vi "Client.vi"() -> ()   [LabVIEW 2021]
uses:
  <vilib>/Utility/file.llb/Write Delimited Spreadsheet (string).vi
panel:
  in  "Electric":dbl
  in  "Smart Home Control":T1(tab)
  out "Boolean":bool
  in  "Username":string
  in  "Password":string
  in  "Login":bool
  in  "AddUser":bool
  in  "DeleteUser":bool
  in  "Logout":bool
  out "Boolean2":bool
  out "LightSensor":bool
  in  "MasterBedroomL1":bool
  in  "MasterBedroomL2":bool
  in  "KitchenToiletL":bool
  in  "KitchenL":bool
  in  "LRToiletL":bool
  in  "LivingRoomL2":bool
  in  "LivingRoomL1":bool
  in  "BalconyL3":bool
  in  "BalconyL2":bool
  in  "BalconyL1":bool
  in  "Bedroom2L":bool
  in  "Bedroom1L":bool
  in  "OffL":bool
  in  "MBToiletDC":bool
  in  "MBToiletDO":bool
  in  "Bedroom2DO":bool
  in  "Bedroom2DC":bool
  out "DoorSensor":bool
  in  "Bedroom1DO":bool
  in  "Bedroom1DC":bool
  in  "MasterBedroomDC":bool
  in  "MasterBedroomDO":bool
  in  "KitchenDO":bool
  in  "KitchenDC":bool
  in  "KitchenToiletDO":bool
  in  "KitchenToiletDC":bool
  in  "LRToiletDC":bool
  in  "LRToiletDO":bool
  in  "LivingRoomDC":bool
  in  "LivingRoomDO":bool
  in  "Balcony2DC":bool
  in  "Balcony2DO":bool
  in  "Balcony1DO1":bool
  in  "Balcony1DC1":bool
  in  "Balcony1DO2":bool
  in  "Balcony1DC2":bool
  in  "OpenD":bool
  in  "CloseD":bool
  in  "MasterBedroomC":dbl(knob) scale=0.0..10.0
  in  "LivingRoomC":dbl(knob) scale=0.0..10.0
  in  "Pause":bool
  in  "Play":bool
  out "TVSensor":bool
  in  "Channel1":bool
  in  "Channel2":bool
  in  "Channel3":bool
  in  "Volume":dbl(knob) scale=0.0..100.0
  in  "Power":bool
  in  "Table Control":string[][](table)
  # "Smart Home Control System"
  # "Off All Lights"
  # "Bedroom 1"
  # "Bedroom 2"
  # "Living Room"
  # "Master Bedroom"
  # "Balcony 1"
  # "Kitchen"
  # "Master Bedroom"
  # "Kitchen"
  # "Living Room"
  # "Toilet"
  # "Toilet"
  # "Toilet"
  # "Bedroom 1"
  # "Balcony 1 to Master"
  # "Balcony 2"
  # "Bedroom 2"
  # "Balcony 1 to Kitchen"
  # "Open All"
  # "Close All"
  # "Master Bedroom"
  # "Living Room"
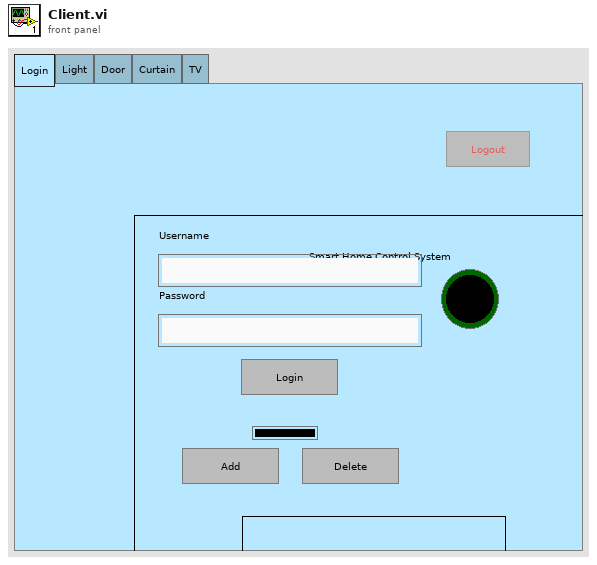
[diagram p1: front panel]
types:
  T1 = enum32{"Login", "Light", "Door", "Curtain", "TV"}
  T2 = enum32{"Page Enabled", "Page Disabled", "Page Disabled & Grayed"}
  T3 = enum8{"Enabled", "Disabled", "Disabled and Grayed Out"}
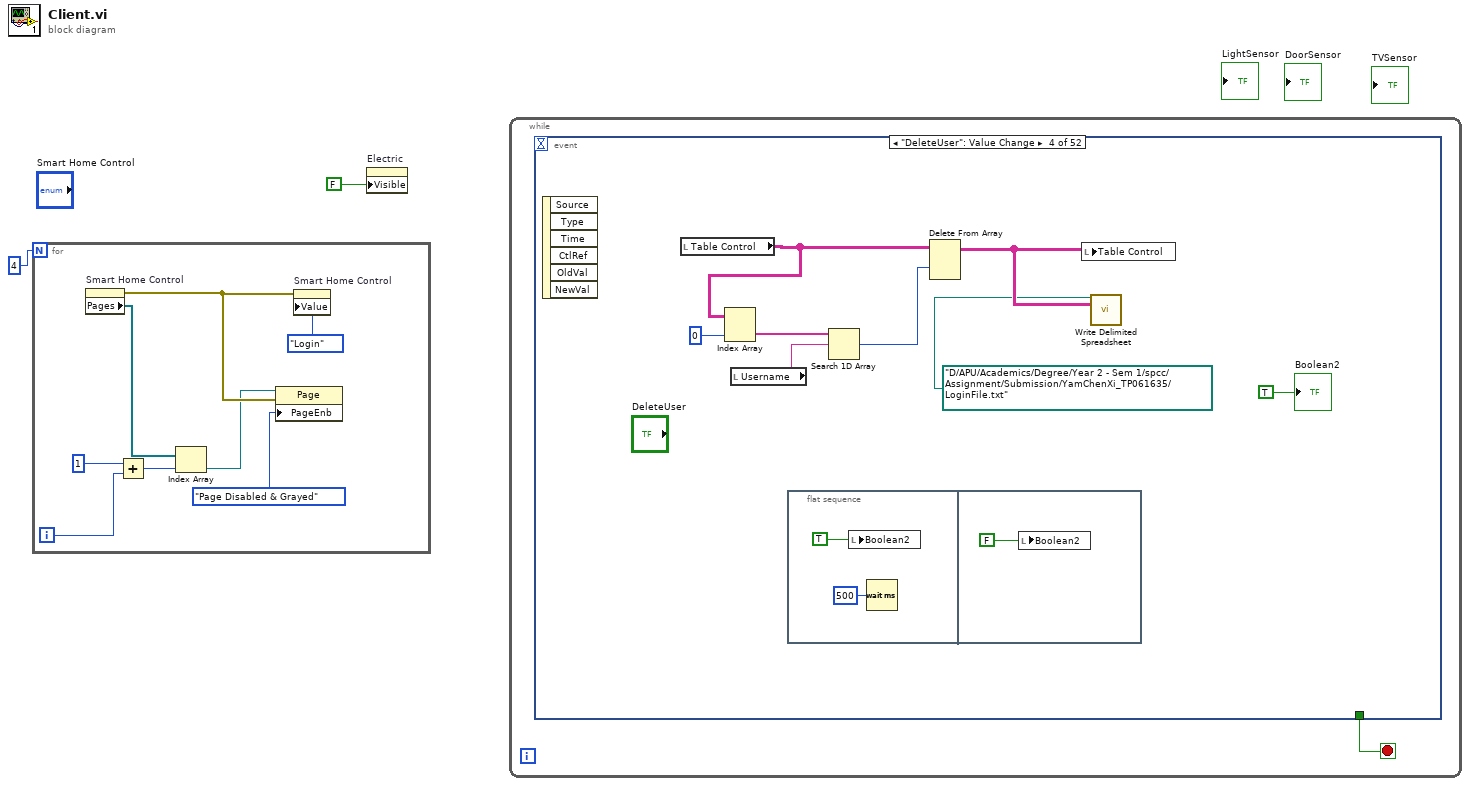
[diagram p0: block diagram]
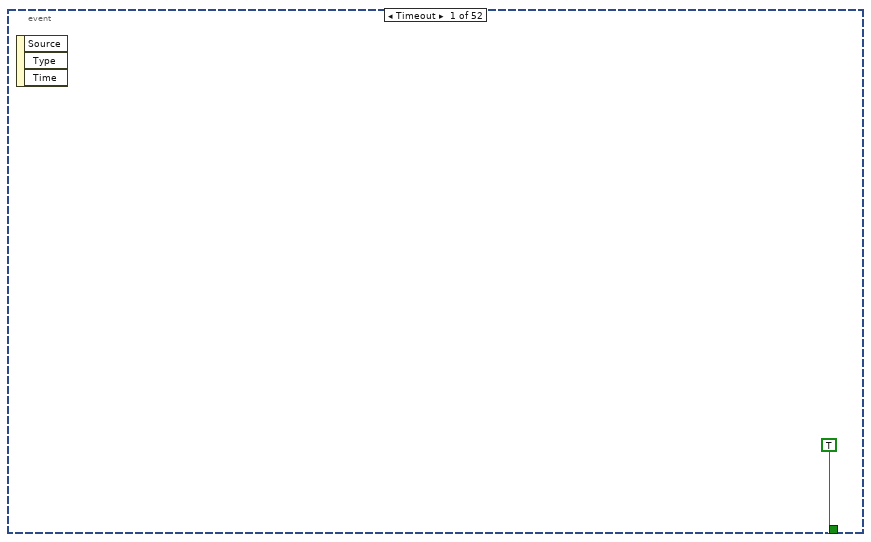
[diagram p2: hidden frame]
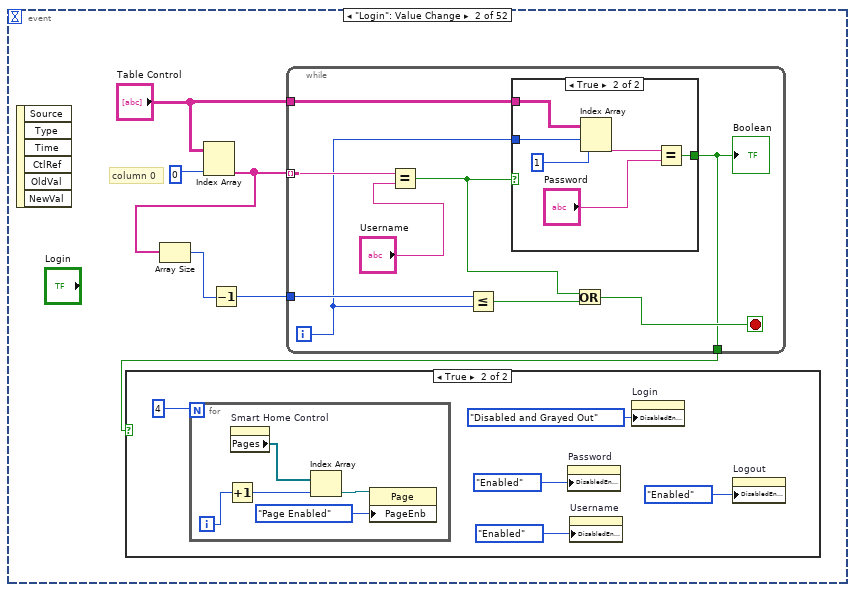
[diagram p3: hidden frame]
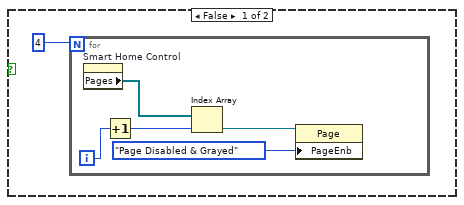
[diagram p4: hidden frame]
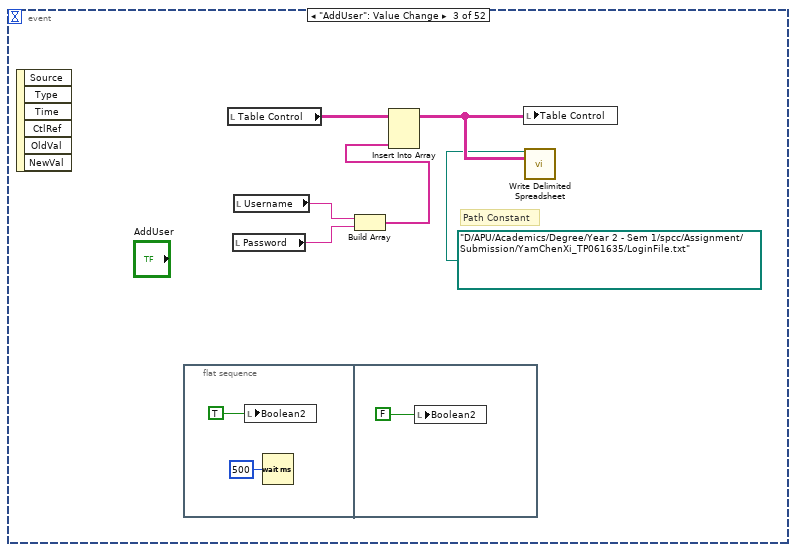
[diagram p6: hidden frame]
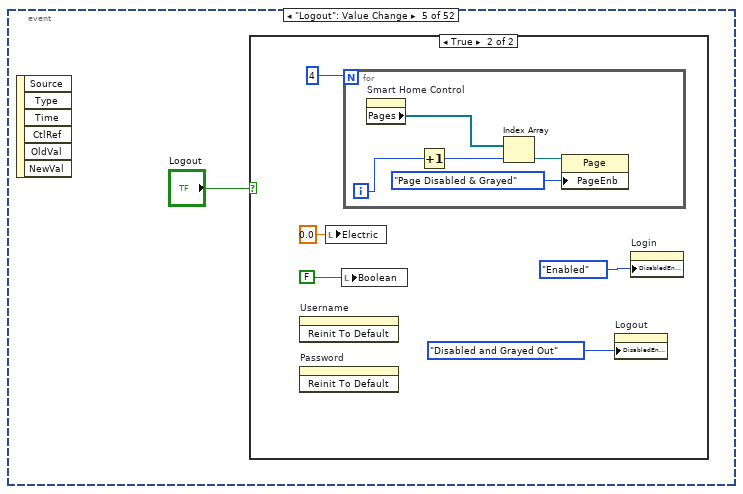
[diagram p7: hidden frame]
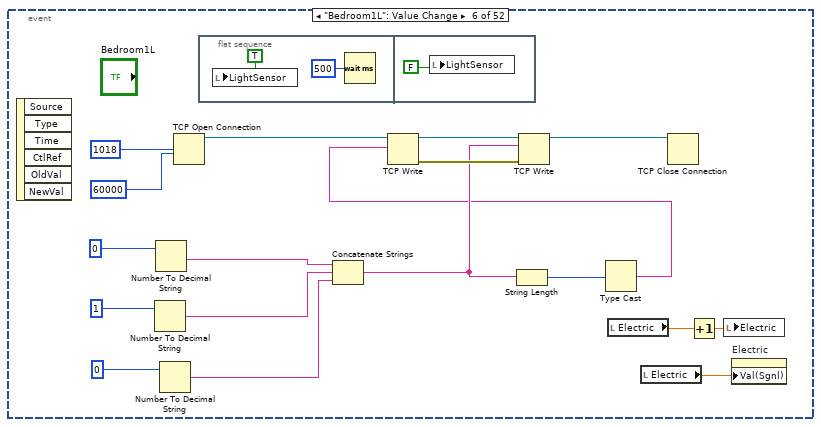
[diagram p9: hidden frame]
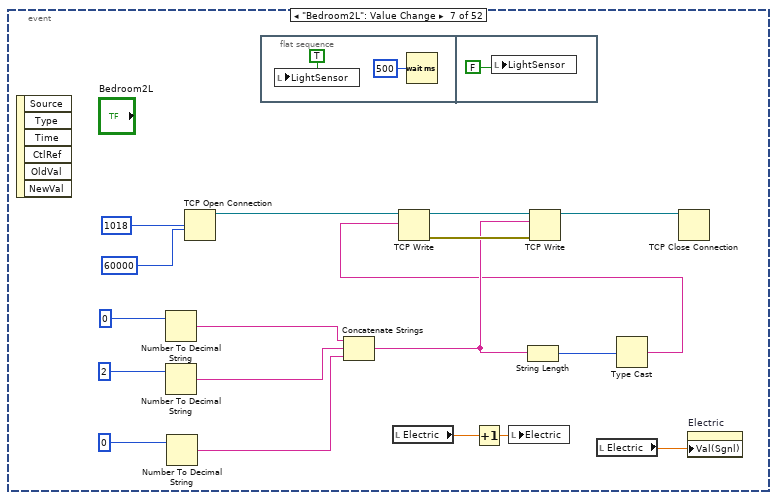
[diagram p10: hidden frame]
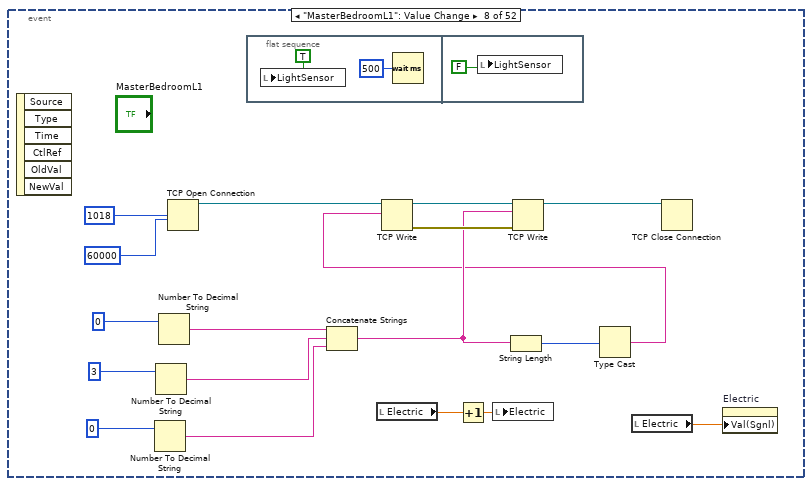
[diagram p11: hidden frame]
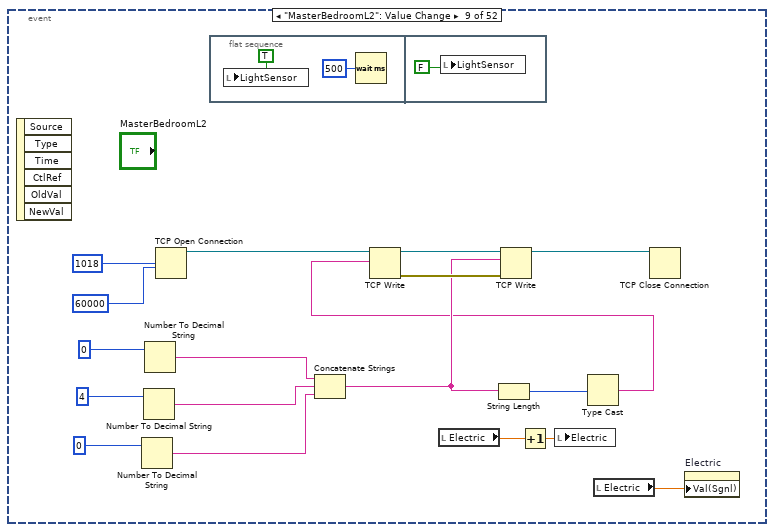
[diagram p12: hidden frame]
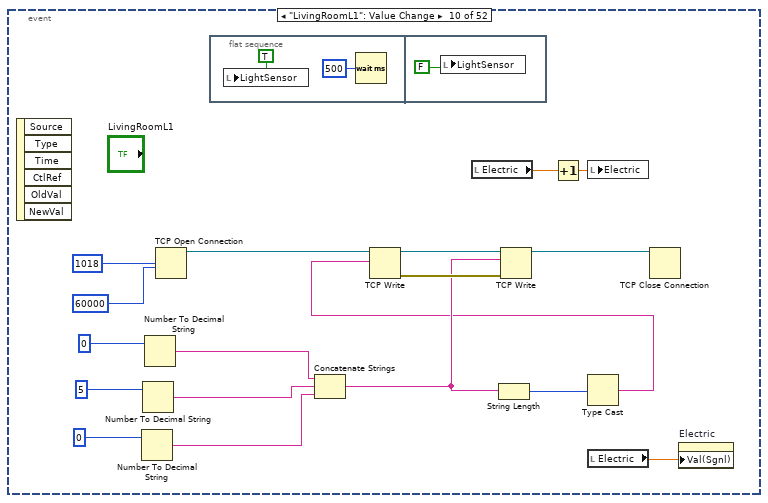
[diagram p13: hidden frame]
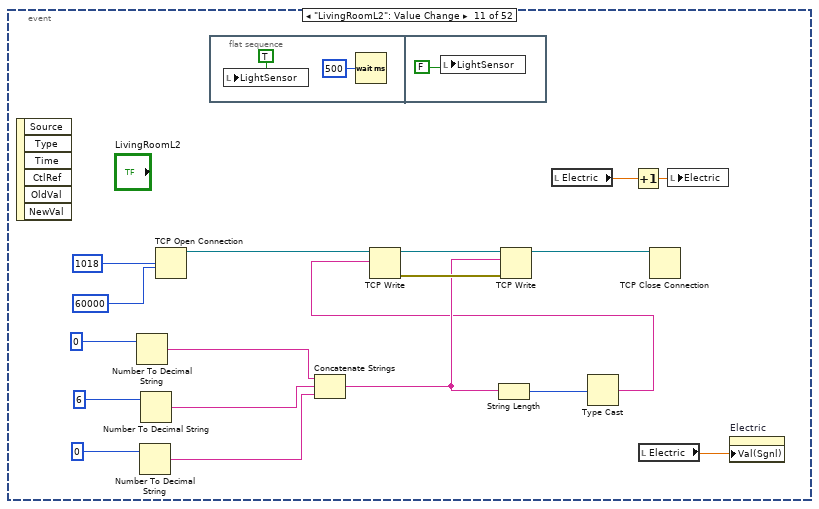
[diagram p14: hidden frame]
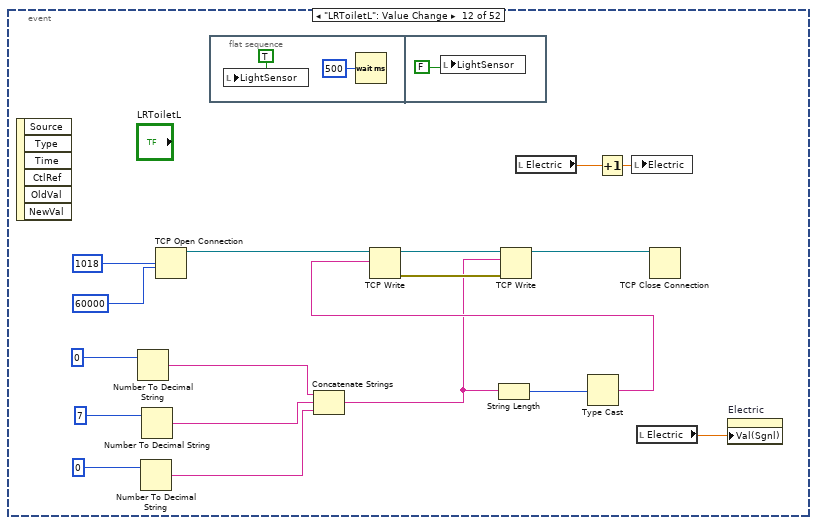
[diagram p15: hidden frame]
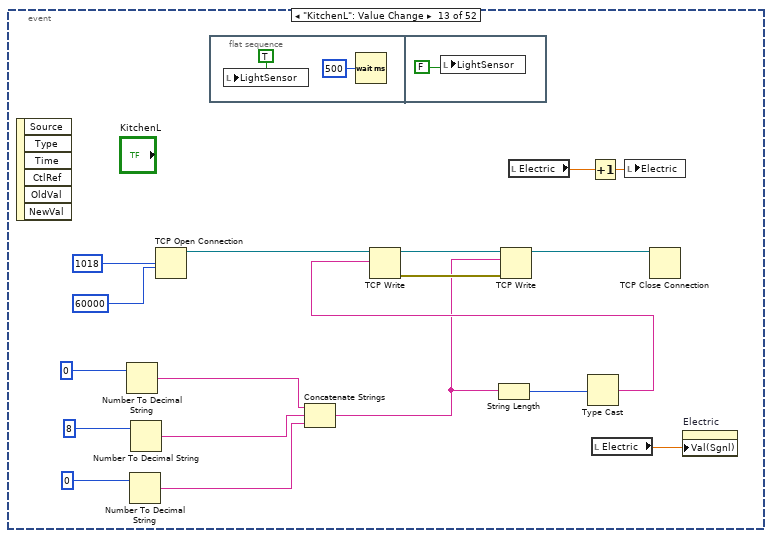
[diagram p16: hidden frame]
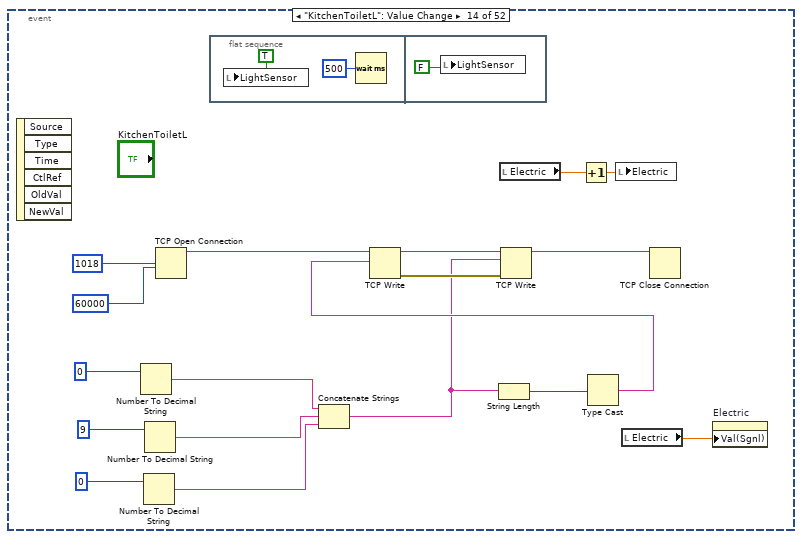
[diagram p17: hidden frame]
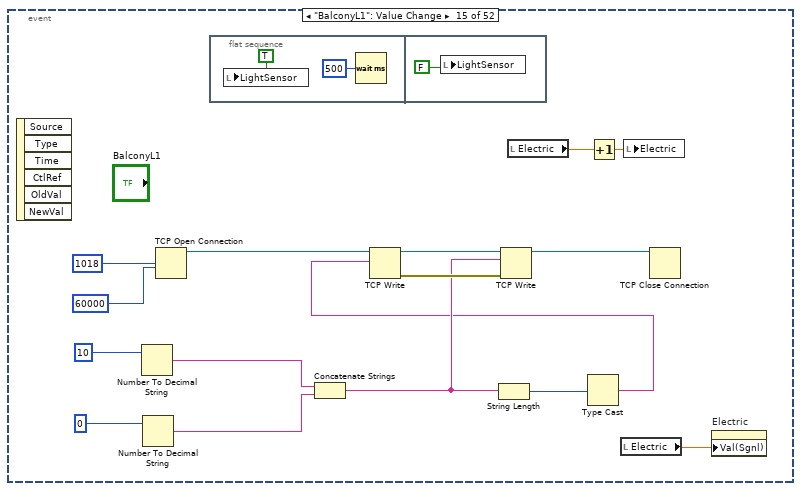
[diagram p18: hidden frame]
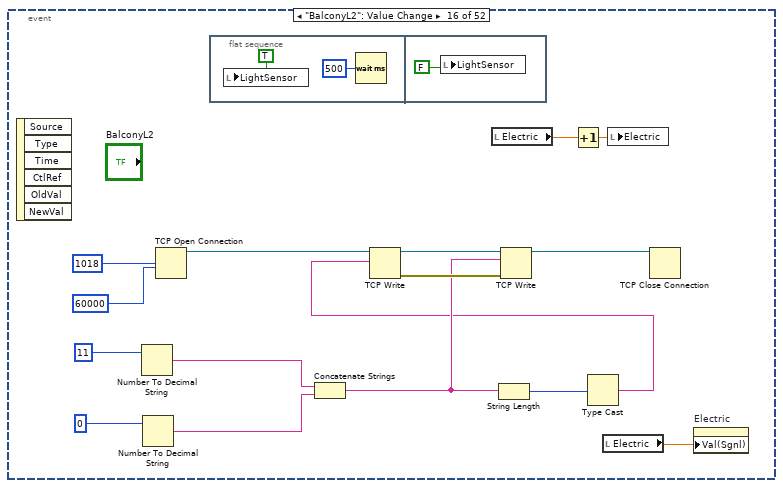
[diagram p19: hidden frame]
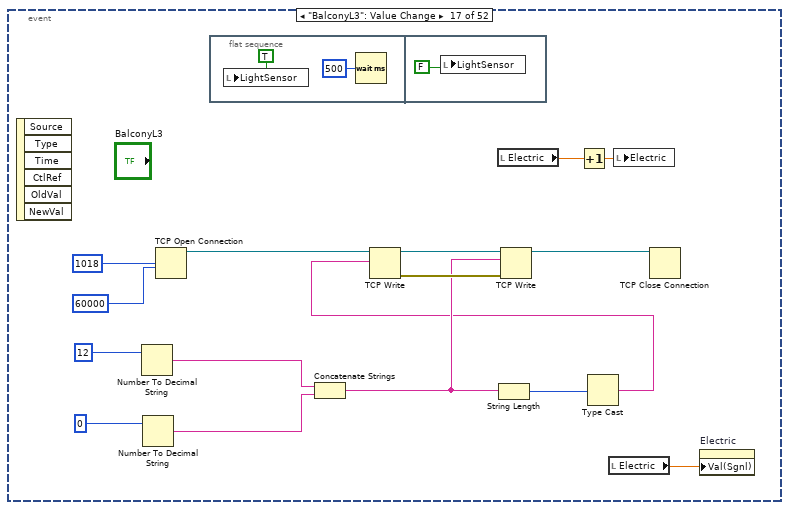
[diagram p20: hidden frame]
diagram:
  n1 = for {
    N: 4 -> [_]
    i -> [w4]
    n2 = property on="Smart Home Control" class="TabCtl (strict)"() -> (error out=w10:errorcluster, "Pages"=w8:refnum<vi>[])  [unwired: 2 in, 1 out]
    n3 = Add(x=1, y=w4) -> (x+y=w6:i32)
    n4 = Index Array "Index Array"(array=w8, index=w6) -> (element=w9:refnum<vi>)
    n5 = property class="Page"(reference=w9, error in=w10, "PageEnb"=T2."Page Disabled & Grayed" ("Page Enabled State")) -> ()  [unwired: 2 out]
    n6 = property on="Smart Home Control" class="TabCtl (strict)"(error in=w10, "Value"=T1."Login" ("Smart Home Control")) -> ()  [unwired: 1 in, 2 out]
  }
  n7 = property on="Electric" class="DigNum (strict)"("Visible"=FALSE) -> ()  [unwired: 2 in, 2 out]
  n8 = while {
    stop <- w11 stop-if-true
    n9 = event shown="[3] \"DeleteUser\": Value Change" {
      selector: _ -> [_ _ _ _ _ _ _ _ _ _ _ _ _ _ _ _ _ _ _ _ _ _ _ _ _ _ _ _ _ _ _ _ _ _ _ _ _ _ _ _ _ _ _ _ _ _ _ _ _ _ _ _]
      dyn-events: _ -> [_ _ _ _ _ _ _ _ _ _ _ _ _ _ _ _ _ _ _ _ _ _ _ _ _ _ _ _ _ _ _ _ _ _ _ _ _ _ _ _ _ _ _ _ _ _ _ _ _ _ _ _]
      timeout: _ -> [_ _ _ _ _ _ _ _ _ _ _ _ _ _ _ _ _ _ _ _ _ _ _ _ _ _ _ _ _ _ _ _ _ _ _ _ _ _ _ _ _ _ _ _ _ _ _ _ _ _ _ _]
      tunnel: [TRUE _ _ _ _ _ _ _ _ _ _ _ _ _ _ _ _ _ _ _ _ _ _ _ _ _ _ _ _ _ _ _ _ _ _ _ _ _ _ _ _ _ _ _ _ _ _ _ _ _ _ _] -> w11
      event Timeout {
        n10 = event-data() -> ()  [unwired: 1 in, 3 out]
      }
      event "Login": Value Change {
        # "column 0"
        n11 = event-data() -> ()  [unwired: 1 in, 6 out]
        n12 = Index Array "Index Array"(array="Table Control", index (col)=0) -> (element=w16:string[])  [unwired: 1 in]
        n13 = Array Size(array=w16) -> (size(s)=w15:i32)
        n14 = Decrement(x=w15) -> (x-1=w14:i32)
        n15 = while {
          tunnel: w16 -> [w43] mode=indexing
          tunnel: "Table Control" -> [w42]
          tunnel: w14 -> [w41]
          tunnel: [w35] -> w13
          i -> [w36]
          stop <- w39 stop-if-true
          n16 = Equal?(x=w43, y="Username") -> (x = y?=w38:bool)
          n17 = Less Or Equal?(x=w41, y=w36) -> (x <= y?=w40:bool)
          n18 = case shown="True" w38 {
            tunnel: w42 -> [_ w49]
            tunnel: [_ w45] -> w35
            tunnel: w36 -> [_ w44]
            frame False {
            }
            frame True {
              n19 = Index Array "Index Array"(array=w49, index (row)=w44, index (col)=1) -> (element=w46:string)
              n20 = Equal?(x=w46, y="Password") -> (x = y?=w45:bool)
            }
          }
          "Boolean" <- w35
          n21 = Or(x=w38, y=w40) -> (x .or. y?=w39:bool)
        }
        n22 = case shown="True" w13 {
          frame False {
            n23 = for {
              N: 4 -> [_]
              i -> [w24]
              n24 = property on="Smart Home Control" class="TabCtl (strict)"() -> ("Pages"=w20:refnum<vi>[])  [unwired: 2 in, 2 out]
              n25 = Increment(x=w24) -> (x+1=w21:i32)
              n26 = Index Array(array=w20, index=w21) -> (element=w23:refnum<vi>)
              n27 = property class="Page"(reference=w23, "PageEnb"=T2."Page Disabled & Grayed" ("Page Enabled State")) -> ()  [unwired: 1 in, 2 out]
            }
          }
          frame True {
            n28 = for {
              N: 4 -> [_]
              i -> [w34]
              n29 = Increment(x=w34) -> (x+1=w30:i32)
              n30 = property on="Smart Home Control" class="TabCtl (strict)"() -> ("Pages"=w32:refnum<vi>[])  [unwired: 2 in, 2 out]
              n31 = Index Array(array=w32, index=w30) -> (element=w33:refnum<vi>)
              n32 = property class="Page"(reference=w33, "PageEnb"=T2."Page Enabled" ("Page Enabled State")) -> ()  [unwired: 1 in, 2 out]
            }
            n33 = property on="Password" class="Str"("DisabledEnum"=T3."Enabled" ("Disabled")) -> ()  [unwired: 2 in, 2 out]
            n34 = property on="Username" class="Str"("DisabledEnum"=T3."Enabled" ("Disabled")) -> ()  [unwired: 2 in, 2 out]
            n35 = property on="Login" class="Bool"("DisabledEnum"=T3."Disabled and Grayed Out" ("Disabled")) -> ()  [unwired: 2 in, 2 out]
            n36 = property on="Logout" class="Bool"("DisabledEnum"=T3."Enabled" ("Disabled")) -> ()  [unwired: 2 in, 2 out]
          }
        }
      }
      event "AddUser": Value Change {
        # "Path Constant"
        n37 = event-data() -> ()  [unwired: 1 in, 6 out]
        n38 = flat-sequence {
          frame #0 {
            n39 = local write "Boolean2"(TRUE) -> ()
            n40 = Wait (ms)(milliseconds to wait=u32 500) -> ()  [unwired: 1 out]
          }
          frame #1 {
            n41 = local write "Boolean2"(FALSE) -> ()
          }
        }
        n42 = local read "Table Control"() -> (w53:string[][])
        n43 = local read "Password"() -> (w54:string)
        n44 = local read "Username"() -> (w55:string)
        n45 = Build Array "Build Array"(w55, w54) -> (w52:string[])
        n46 = Insert Into Array "Insert Into Array"(array=w53, new element=w52) -> (w51:string[][])  [unwired: 2 in]
        n47 = local write "Table Control"(w51) -> ()
        n48 = call-poly <vilib>:"Write Delimited Spreadsheet.vi"("file path (dialog if empty)"=path "D:/APU/Academics/Degree/Year 2 - Sem 1/spcc/Assignment/Submission/YamChenXi_TP061635/LoginFile.txt", "2D data"=w51) -> ()  [unwired: 12 in, 2 out]
      }
      event "DeleteUser": Value Change {
        n49 = event-data() -> ()  [unwired: 1 in, 6 out]
        n50 = local read "Table Control"() -> (w66:string[][])
        n51 = Index Array "Index Array"(array=w66, index (col)=0) -> (element=w64:string[])  [unwired: 1 in]
        n52 = local read "Username"() -> (w63:string)
        n53 = flat-sequence {
          frame #0 {
            n54 = local write "Boolean2"(TRUE) -> ()
            n55 = Wait (ms)(milliseconds to wait=u32 500) -> ()  [unwired: 1 out]
          }
          frame #1 {
            n56 = local write "Boolean2"(FALSE) -> ()
          }
        }
        n57 = Search 1D Array(1D array=w64, element=w63) -> (index of element=w62:i32)  [unwired: 1 in]
        n58 = Delete From Array "Delete From Array"(array=w66, index (row)=w62) -> (array with subset deleted=w61:string[][])  [unwired: 2 in, 1 out]
        n59 = local write "Table Control"(w61) -> ()
        n60 = call-poly <vilib>:"Write Delimited Spreadsheet.vi"("file path (dialog if empty)"=path "D:/APU/Academics/Degree/Year 2 - Sem 1/spcc/Assignment/Submission/YamChenXi_TP061635/LoginFile.txt", "2D data"=w61) -> ()  [unwired: 12 in, 2 out]
        "Boolean2" <- TRUE
      }
      event "Logout": Value Change {
        n61 = event-data() -> ()  [unwired: 1 in, 6 out]
        n62 = case shown="True" "Logout" {
          frame False {
          }
          frame True {
            n63 = invoke on="Username" class="Str" method="Reinit To Default"() -> ()  [unwired: 3 in, 3 out]
            n64 = invoke on="Password" class="Str" method="Reinit To Default"() -> ()  [unwired: 3 in, 3 out]
            n65 = local write "Electric"(0.0 ("Electric")) -> ()
            n66 = local write "Boolean"(FALSE) -> ()
            n67 = for {
              N: 4 -> [_]
              i -> [w80]
              n68 = property on="Smart Home Control" class="TabCtl (strict)"() -> ("Pages"=w76:refnum<vi>[])  [unwired: 2 in, 2 out]
              n69 = Increment(x=w80) -> (x+1=w77:i32)
              n70 = Index Array(array=w76, index=w77) -> (element=w79:refnum<vi>)
              n71 = property class="Page"(reference=w79, "PageEnb"=T2."Page Disabled & Grayed" ("Page Enabled State")) -> ()  [unwired: 1 in, 2 out]
            }
            n72 = property on="Logout" class="Bool"("DisabledEnum"=T3."Disabled and Grayed Out" ("Disabled")) -> ()  [unwired: 2 in, 2 out]
            n73 = property on="Login" class="Bool"("DisabledEnum"=T3."Enabled" ("Disabled")) -> ()  [unwired: 2 in, 2 out]
          }
        }
      }
      event "Bedroom1L": Value Change {
        n74 = event-data() -> ()  [unwired: 1 in, 6 out]
        n75 = Number To Decimal String(number=1) -> (decimal integer string=w92:string)  [unwired: 1 in]
        n76 = Number To Decimal String(number=0) -> (decimal integer string=w86:string)  [unwired: 1 in]
        n77 = Number To Decimal String(number=0) -> (decimal integer string=w93:string)  [unwired: 1 in]
        n78 = TCP Open Connection(remote port or service name=1018, timeout ms (60000)=60000) -> (connection ID=w96:refnum<k5>)  [unwired: 3 in, 1 out]
        n79 = flat-sequence {
          frame #0 {
            n80 = local write "LightSensor"(TRUE) -> ()
            n81 = Wait (ms)(milliseconds to wait=u32 500) -> ()  [unwired: 1 out]
          }
          frame #1 {
            n82 = local write "LightSensor"(FALSE) -> ()
          }
        }
        n83 = Concatenate Strings "Concatenate Strings"(w86, w92, w93) -> (w85:string)
        n84 = String Length(string=w85) -> (length=w94:i32)
        n85 = Type Cast(x=w94) -> (*(type *) &x=w81:string)  [unwired: 1 in]
        n86 = TCP Write(connection ID=w96, data in=w81) -> (connection ID out=w97:refnum<k5>, error out=w95:errorcluster)  [unwired: 2 in, 1 out]
        n87 = TCP Write(connection ID=w97, data in=w85, error in (no error)=w95) -> (connection ID out=w98:refnum<k5>)  [unwired: 1 in, 2 out]
        n88 = local read "Electric"() -> (w83:dbl)
        n89 = local read "Electric"() -> (w82:dbl)
        n90 = TCP Close Connection(connection ID=w98) -> ()  [unwired: 2 in, 2 out]
        n91 = Increment(x=w83) -> (x+1=w84:dbl)
        n92 = local write "Electric"(w84) -> ()
        n93 = property on="Electric" class="DigNum (strict)"("Val(Sgnl)"=w82) -> ()  [unwired: 2 in, 2 out]
      }
      event "Bedroom2L": Value Change {
        n94 = event-data() -> ()  [unwired: 1 in, 6 out]
        n95 = Number To Decimal String(number=0) -> (decimal integer string=w105:string)  [unwired: 1 in]
        n96 = Number To Decimal String(number=2) -> (decimal integer string=w107:string)  [unwired: 1 in]
        n97 = Number To Decimal String(number=0) -> (decimal integer string=w114:string)  [unwired: 1 in]
        n98 = TCP Open Connection(remote port or service name=1018, timeout ms (60000)=60000) -> (connection ID=w117:refnum<k5>)  [unwired: 3 in, 1 out]
        n99 = flat-sequence {
          frame #0 {
            n100 = local write "LightSensor"(TRUE) -> ()
            n101 = Wait (ms)(milliseconds to wait=u32 500) -> ()  [unwired: 1 out]
          }
          frame #1 {
            n102 = local write "LightSensor"(FALSE) -> ()
          }
        }
        n103 = Concatenate Strings "Concatenate Strings"(w105, w107, w114) -> (w109:string)
        n104 = local read "Electric"() -> (w103:dbl)
        n105 = Increment(x=w103) -> (x+1=w104:dbl)
        n106 = local write "Electric"(w104) -> ()
        n107 = String Length(string=w109) -> (length=w115:i32)
        n108 = local read "Electric"() -> (w102:dbl)
        n109 = Type Cast(x=w115) -> (*(type *) &x=w108:string)  [unwired: 1 in]
        n110 = TCP Write(connection ID=w117, data in=w108) -> (connection ID out=w118:refnum<k5>, error out=w116:errorcluster)  [unwired: 2 in, 1 out]
        n111 = TCP Write(connection ID=w118, data in=w109, error in (no error)=w116) -> (connection ID out=w119:refnum<k5>)  [unwired: 1 in, 2 out]
        n112 = TCP Close Connection(connection ID=w119) -> ()  [unwired: 2 in, 2 out]
        n113 = property on="Electric" class="DigNum (strict)"("Val(Sgnl)"=w102) -> ()  [unwired: 2 in, 2 out]
      }
      event "MasterBedroomL1": Value Change {
        n114 = event-data() -> ()  [unwired: 1 in, 6 out]
        n115 = Number To Decimal String(number=0) -> (decimal integer string=w135:string)  [unwired: 1 in]
        n116 = Number To Decimal String(number=3) -> (decimal integer string=w134:string)  [unwired: 1 in]
        n117 = Number To Decimal String(number=0) -> (decimal integer string=w126:string)  [unwired: 1 in]
        n118 = TCP Open Connection(remote port or service name=1018, timeout ms (60000)=60000) -> (connection ID=w138:refnum<k5>)  [unwired: 3 in, 1 out]
        n119 = flat-sequence {
          frame #0 {
            n120 = local write "LightSensor"(TRUE) -> ()
            n121 = Wait (ms)(milliseconds to wait=u32 500) -> ()  [unwired: 1 out]
          }
          frame #1 {
            n122 = local write "LightSensor"(FALSE) -> ()
          }
        }
        n123 = Concatenate Strings "Concatenate Strings"(w126, w134, w135) -> (w129:string)
        n124 = local read "Electric"() -> (w124:dbl)
        n125 = Increment(x=w124) -> (x+1=w125:dbl)
        n126 = local write "Electric"(w125) -> ()
        n127 = String Length(string=w129) -> (length=w136:i32)
        n128 = Type Cast(x=w136) -> (*(type *) &x=w128:string)  [unwired: 1 in]
        n129 = TCP Write(connection ID=w138, data in=w128) -> (connection ID out=w139:refnum<k5>, error out=w137:errorcluster)  [unwired: 2 in, 1 out]
        n130 = TCP Write(connection ID=w139, data in=w129, error in (no error)=w137) -> (connection ID out=w140:refnum<k5>)  [unwired: 1 in, 2 out]
        n131 = local read "Electric"() -> (w123:dbl)
        n132 = TCP Close Connection(connection ID=w140) -> ()  [unwired: 2 in, 2 out]
        n133 = property on="Electric" class="DigNum (strict)"("Val(Sgnl)"=w123) -> ()  [unwired: 2 in, 2 out]
      }
      event "MasterBedroomL2": Value Change {
        n134 = event-data() -> ()  [unwired: 1 in, 6 out]
        n135 = Number To Decimal String(number=0) -> (decimal integer string=w156:string)  [unwired: 1 in]
        n136 = Number To Decimal String(number=4) -> (decimal integer string=w155:string)  [unwired: 1 in]
        n137 = Number To Decimal String(number=0) -> (decimal integer string=w147:string)  [unwired: 1 in]
        n138 = TCP Open Connection(remote port or service name=1018, timeout ms (60000)=60000) -> (connection ID=w159:refnum<k5>)  [unwired: 3 in, 1 out]
        n139 = flat-sequence {
          frame #0 {
            n140 = local write "LightSensor"(TRUE) -> ()
            n141 = Wait (ms)(milliseconds to wait=u32 500) -> ()  [unwired: 1 out]
          }
          frame #1 {
            n142 = local write "LightSensor"(FALSE) -> ()
          }
        }
        n143 = Concatenate Strings "Concatenate Strings"(w147, w155, w156) -> (w150:string)
        n144 = local read "Electric"() -> (w146:dbl)
        n145 = String Length(string=w150) -> (length=w157:i32)
        n146 = Increment(x=w146) -> (x+1=w145:dbl)
        n147 = local write "Electric"(w145) -> ()
        n148 = Type Cast(x=w157) -> (*(type *) &x=w149:string)  [unwired: 1 in]
        n149 = TCP Write(connection ID=w159, data in=w149) -> (connection ID out=w160:refnum<k5>, error out=w158:errorcluster)  [unwired: 2 in, 1 out]
        n150 = TCP Write(connection ID=w160, data in=w150, error in (no error)=w158) -> (connection ID out=w161:refnum<k5>)  [unwired: 1 in, 2 out]
        n151 = local read "Electric"() -> (w144:dbl)
        n152 = TCP Close Connection(connection ID=w161) -> ()  [unwired: 2 in, 2 out]
        n153 = property on="Electric" class="DigNum (strict)"("Val(Sgnl)"=w144) -> ()  [unwired: 2 in, 2 out]
      }
      event "LivingRoomL1": Value Change {
        n154 = event-data() -> ()  [unwired: 1 in, 6 out]
        n155 = Number To Decimal String(number=0) -> (decimal integer string=w177:string)  [unwired: 1 in]
        n156 = Number To Decimal String(number=5) -> (decimal integer string=w176:string)  [unwired: 1 in]
        n157 = Number To Decimal String(number=0) -> (decimal integer string=w168:string)  [unwired: 1 in]
        n158 = TCP Open Connection(remote port or service name=1018, timeout ms (60000)=60000) -> (connection ID=w180:refnum<k5>)  [unwired: 3 in, 1 out]
        n159 = flat-sequence {
          frame #0 {
            n160 = local write "LightSensor"(TRUE) -> ()
            n161 = Wait (ms)(milliseconds to wait=u32 500) -> ()  [unwired: 1 out]
          }
          frame #1 {
            n162 = local write "LightSensor"(FALSE) -> ()
          }
        }
        n163 = Concatenate Strings "Concatenate Strings"(w168, w176, w177) -> (w171:string)
        n164 = local read "Electric"() -> (w167:dbl)
        n165 = String Length(string=w171) -> (length=w178:i32)
        n166 = Increment(x=w167) -> (x+1=w166:dbl)
        n167 = local write "Electric"(w166) -> ()
        n168 = Type Cast(x=w178) -> (*(type *) &x=w170:string)  [unwired: 1 in]
        n169 = TCP Write(connection ID=w180, data in=w170) -> (connection ID out=w181:refnum<k5>, error out=w179:errorcluster)  [unwired: 2 in, 1 out]
        n170 = TCP Write(connection ID=w181, data in=w171, error in (no error)=w179) -> (connection ID out=w182:refnum<k5>)  [unwired: 1 in, 2 out]
        n171 = local read "Electric"() -> (w165:dbl)
        n172 = TCP Close Connection(connection ID=w182) -> ()  [unwired: 2 in, 2 out]
        n173 = property on="Electric" class="DigNum (strict)"("Val(Sgnl)"=w165) -> ()  [unwired: 2 in, 2 out]
      }
      event "LivingRoomL2": Value Change {
        n174 = event-data() -> ()  [unwired: 1 in, 6 out]
        n175 = Number To Decimal String(number=0) -> (decimal integer string=w189:string)  [unwired: 1 in]
        n176 = Number To Decimal String(number=0) -> (decimal integer string=w198:string)  [unwired: 1 in]
        n177 = Number To Decimal String(number=6) -> (decimal integer string=w197:string)  [unwired: 1 in]
        n178 = TCP Open Connection(remote port or service name=1018, timeout ms (60000)=60000) -> (connection ID=w201:refnum<k5>)  [unwired: 3 in, 1 out]
        n179 = flat-sequence {
          frame #0 {
            n180 = local write "LightSensor"(TRUE) -> ()
            n181 = Wait (ms)(milliseconds to wait=u32 500) -> ()  [unwired: 1 out]
          }
          frame #1 {
            n182 = local write "LightSensor"(FALSE) -> ()
          }
        }
        n183 = Concatenate Strings "Concatenate Strings"(w189, w197, w198) -> (w192:string)
        n184 = String Length(string=w192) -> (length=w199:i32)
        n185 = local read "Electric"() -> (w188:dbl)
        n186 = Type Cast(x=w199) -> (*(type *) &x=w191:string)  [unwired: 1 in]
        n187 = TCP Write(connection ID=w201, data in=w191) -> (connection ID out=w202:refnum<k5>, error out=w200:errorcluster)  [unwired: 2 in, 1 out]
        n188 = TCP Write(connection ID=w202, data in=w192, error in (no error)=w200) -> (connection ID out=w203:refnum<k5>)  [unwired: 1 in, 2 out]
        n189 = Increment(x=w188) -> (x+1=w187:dbl)
        n190 = local read "Electric"() -> (w186:dbl)
        n191 = TCP Close Connection(connection ID=w203) -> ()  [unwired: 2 in, 2 out]
        n192 = local write "Electric"(w187) -> ()
        n193 = property on="Electric" class="DigNum (strict)"("Val(Sgnl)"=w186) -> ()  [unwired: 2 in, 2 out]
      }
      event "LRToiletL": Value Change {
        n194 = event-data() -> ()  [unwired: 1 in, 6 out]
        n195 = Number To Decimal String(number=0) -> (decimal integer string=w211:string)  [unwired: 1 in]
        n196 = Number To Decimal String(number=0) -> (decimal integer string=w216:string)  [unwired: 1 in]
        n197 = Number To Decimal String(number=7) -> (decimal integer string=w215:string)  [unwired: 1 in]
        n198 = TCP Open Connection(remote port or service name=1018, timeout ms (60000)=60000) -> (connection ID=w222:refnum<k5>)  [unwired: 3 in, 1 out]
        n199 = flat-sequence {
          frame #0 {
            n200 = local write "LightSensor"(TRUE) -> ()
            n201 = Wait (ms)(milliseconds to wait=u32 500) -> ()  [unwired: 1 out]
          }
          frame #1 {
            n202 = local write "LightSensor"(FALSE) -> ()
          }
        }
        n203 = Concatenate Strings "Concatenate Strings"(w211, w215, w216) -> (w210:string)
        n204 = String Length(string=w210) -> (length=w220:i32)
        n205 = local read "Electric"() -> (w209:dbl)
        n206 = Type Cast(x=w220) -> (*(type *) &x=w217:string)  [unwired: 1 in]
        n207 = TCP Write(connection ID=w222, data in=w217) -> (connection ID out=w223:refnum<k5>, error out=w221:errorcluster)  [unwired: 2 in, 1 out]
        n208 = TCP Write(connection ID=w223, data in=w210, error in (no error)=w221) -> (connection ID out=w224:refnum<k5>)  [unwired: 1 in, 2 out]
        n209 = Increment(x=w209) -> (x+1=w208:dbl)
        n210 = local write "Electric"(w208) -> ()
        n211 = local read "Electric"() -> (w207:dbl)
        n212 = TCP Close Connection(connection ID=w224) -> ()  [unwired: 2 in, 2 out]
        n213 = property on="Electric" class="DigNum (strict)"("Val(Sgnl)"=w207) -> ()  [unwired: 2 in, 2 out]
      }
      event "KitchenL": Value Change {
        n214 = event-data() -> ()  [unwired: 1 in, 6 out]
        n215 = Number To Decimal String(number=0) -> (decimal integer string=w232:string)  [unwired: 1 in]
        n216 = Number To Decimal String(number=0) -> (decimal integer string=w237:string)  [unwired: 1 in]
        n217 = Number To Decimal String(number=8) -> (decimal integer string=w236:string)  [unwired: 1 in]
        n218 = TCP Open Connection(remote port or service name=1018, timeout ms (60000)=60000) -> (connection ID=w243:refnum<k5>)  [unwired: 3 in, 1 out]
        n219 = flat-sequence {
          frame #0 {
            n220 = local write "LightSensor"(TRUE) -> ()
            n221 = Wait (ms)(milliseconds to wait=u32 500) -> ()  [unwired: 1 out]
          }
          frame #1 {
            n222 = local write "LightSensor"(FALSE) -> ()
          }
        }
        n223 = Concatenate Strings "Concatenate Strings"(w232, w236, w237) -> (w231:string)
        n224 = String Length(string=w231) -> (length=w241:i32)
        n225 = local read "Electric"() -> (w230:dbl)
        n226 = Type Cast(x=w241) -> (*(type *) &x=w238:string)  [unwired: 1 in]
        n227 = TCP Write(connection ID=w243, data in=w238) -> (connection ID out=w244:refnum<k5>, error out=w242:errorcluster)  [unwired: 2 in, 1 out]
        n228 = TCP Write(connection ID=w244, data in=w231, error in (no error)=w242) -> (connection ID out=w245:refnum<k5>)  [unwired: 1 in, 2 out]
        n229 = Increment(x=w230) -> (x+1=w229:dbl)
        n230 = local read "Electric"() -> (w228:dbl)
        n231 = local write "Electric"(w229) -> ()
        n232 = TCP Close Connection(connection ID=w245) -> ()  [unwired: 2 in, 2 out]
        n233 = property on="Electric" class="DigNum (strict)"("Val(Sgnl)"=w228) -> ()  [unwired: 2 in, 2 out]
      }
      event "KitchenToiletL": Value Change {
        n234 = event-data() -> ()  [unwired: 1 in, 6 out]
        n235 = Number To Decimal String(number=0) -> (decimal integer string=w253:string)  [unwired: 1 in]
        n236 = Number To Decimal String(number=0) -> (decimal integer string=w258:string)  [unwired: 1 in]
        n237 = Number To Decimal String(number=9) -> (decimal integer string=w257:string)  [unwired: 1 in]
        n238 = TCP Open Connection(remote port or service name=1018, timeout ms (60000)=60000) -> (connection ID=w264:refnum<k5>)  [unwired: 3 in, 1 out]
        n239 = flat-sequence {
          frame #0 {
            n240 = local write "LightSensor"(TRUE) -> ()
            n241 = Wait (ms)(milliseconds to wait=u32 500) -> ()  [unwired: 1 out]
          }
          frame #1 {
            n242 = local write "LightSensor"(FALSE) -> ()
          }
        }
        n243 = Concatenate Strings "Concatenate Strings"(w253, w257, w258) -> (w252:string)
        n244 = String Length(string=w252) -> (length=w262:i32)
        n245 = local read "Electric"() -> (w251:dbl)
        n246 = Increment(x=w251) -> (x+1=w250:dbl)
        n247 = Type Cast(x=w262) -> (*(type *) &x=w259:string)  [unwired: 1 in]
        n248 = TCP Write(connection ID=w264, data in=w259) -> (connection ID out=w265:refnum<k5>, error out=w263:errorcluster)  [unwired: 2 in, 1 out]
        n249 = TCP Write(connection ID=w265, data in=w252, error in (no error)=w263) -> (connection ID out=w266:refnum<k5>)  [unwired: 1 in, 2 out]
        n250 = local write "Electric"(w250) -> ()
        n251 = local read "Electric"() -> (w249:dbl)
        n252 = TCP Close Connection(connection ID=w266) -> ()  [unwired: 2 in, 2 out]
        n253 = property on="Electric" class="DigNum (strict)"("Val(Sgnl)"=w249) -> ()  [unwired: 2 in, 2 out]
      }
      event "BalconyL1": Value Change {
        n254 = event-data() -> ()  [unwired: 1 in, 6 out]
        n255 = Number To Decimal String(number=10) -> (decimal integer string=w279:string)  [unwired: 1 in]
        n256 = Number To Decimal String(number=0) -> (decimal integer string=w280:string)  [unwired: 1 in]
        n257 = TCP Open Connection(remote port or service name=1018, timeout ms (60000)=60000) -> (connection ID=w283:refnum<k5>)  [unwired: 3 in, 1 out]
        n258 = flat-sequence {
          frame #0 {
            n259 = local write "LightSensor"(TRUE) -> ()
            n260 = Wait (ms)(milliseconds to wait=u32 500) -> ()  [unwired: 1 out]
          }
          frame #1 {
            n261 = local write "LightSensor"(FALSE) -> ()
          }
        }
        n262 = Concatenate Strings "Concatenate Strings"(w279, w280) -> (w274:string)
        n263 = String Length(string=w274) -> (length=w281:i32)
        n264 = local read "Electric"() -> (w272:dbl)
        n265 = Type Cast(x=w281) -> (*(type *) &x=w273:string)  [unwired: 1 in]
        n266 = TCP Write(connection ID=w283, data in=w273) -> (connection ID out=w284:refnum<k5>, error out=w282:errorcluster)  [unwired: 2 in, 1 out]
        n267 = TCP Write(connection ID=w284, data in=w274, error in (no error)=w282) -> (connection ID out=w285:refnum<k5>)  [unwired: 1 in, 2 out]
        n268 = Increment(x=w272) -> (x+1=w271:dbl)
        n269 = local read "Electric"() -> (w270:dbl)
        n270 = local write "Electric"(w271) -> ()
        n271 = TCP Close Connection(connection ID=w285) -> ()  [unwired: 2 in, 2 out]
        n272 = property on="Electric" class="DigNum (strict)"("Val(Sgnl)"=w270) -> ()  [unwired: 2 in, 2 out]
      }
      event "BalconyL2": Value Change {
        n273 = event-data() -> ()  [unwired: 1 in, 6 out]
        n274 = Number To Decimal String(number=11) -> (decimal integer string=w298:string)  [unwired: 1 in]
        n275 = Number To Decimal String(number=0) -> (decimal integer string=w299:string)  [unwired: 1 in]
        n276 = TCP Open Connection(remote port or service name=1018, timeout ms (60000)=60000) -> (connection ID=w302:refnum<k5>)  [unwired: 3 in, 1 out]
        n277 = flat-sequence {
          frame #0 {
            n278 = local write "LightSensor"(TRUE) -> ()
            n279 = Wait (ms)(milliseconds to wait=u32 500) -> ()  [unwired: 1 out]
          }
          frame #1 {
            n280 = local write "LightSensor"(FALSE) -> ()
          }
        }
        n281 = Concatenate Strings "Concatenate Strings"(w298, w299) -> (w293:string)
        n282 = local read "Electric"() -> (w291:dbl)
        n283 = String Length(string=w293) -> (length=w300:i32)
        n284 = Increment(x=w291) -> (x+1=w290:dbl)
        n285 = Type Cast(x=w300) -> (*(type *) &x=w292:string)  [unwired: 1 in]
        n286 = TCP Write(connection ID=w302, data in=w292) -> (connection ID out=w303:refnum<k5>, error out=w301:errorcluster)  [unwired: 2 in, 1 out]
        n287 = TCP Write(connection ID=w303, data in=w293, error in (no error)=w301) -> (connection ID out=w304:refnum<k5>)  [unwired: 1 in, 2 out]
        n288 = local read "Electric"() -> (w289:dbl)
        n289 = local write "Electric"(w290) -> ()
        n290 = TCP Close Connection(connection ID=w304) -> ()  [unwired: 2 in, 2 out]
        n291 = property on="Electric" class="DigNum (strict)"("Val(Sgnl)"=w289) -> ()  [unwired: 2 in, 2 out]
      }
      event "BalconyL3": Value Change {
        n292 = event-data() -> ()  [unwired: 1 in, 6 out]
        n293 = Number To Decimal String(number=12) -> (decimal integer string=w317:string)  [unwired: 1 in]
        n294 = Number To Decimal String(number=0) -> (decimal integer string=w318:string)  [unwired: 1 in]
        n295 = TCP Open Connection(remote port or service name=1018, timeout ms (60000)=60000) -> (connection ID=w321:refnum<k5>)  [unwired: 3 in, 1 out]
        n296 = flat-sequence {
          frame #0 {
            n297 = local write "LightSensor"(TRUE) -> ()
            n298 = Wait (ms)(milliseconds to wait=u32 500) -> ()  [unwired: 1 out]
          }
          frame #1 {
            n299 = local write "LightSensor"(FALSE) -> ()
          }
        }
        n300 = Concatenate Strings "Concatenate Strings"(w317, w318) -> (w312:string)
        n301 = local read "Electric"() -> (w310:dbl)
        n302 = String Length(string=w312) -> (length=w319:i32)
        n303 = Increment(x=w310) -> (x+1=w309:dbl)
        n304 = Type Cast(x=w319) -> (*(type *) &x=w311:string)  [unwired: 1 in]
        n305 = TCP Write(connection ID=w321, data in=w311) -> (connection ID out=w322:refnum<k5>, error out=w320:errorcluster)  [unwired: 2 in, 1 out]
        n306 = TCP Write(connection ID=w322, data in=w312, error in (no error)=w320) -> (connection ID out=w323:refnum<k5>)  [unwired: 1 in, 2 out]
        n307 = local read "Electric"() -> (w308:dbl)
        n308 = local write "Electric"(w309) -> ()
        n309 = TCP Close Connection(connection ID=w323) -> ()  [unwired: 2 in, 2 out]
        n310 = property on="Electric" class="DigNum (strict)"("Val(Sgnl)"=w308) -> ()  [unwired: 2 in, 2 out]
      }
      event "OffL": Value Change {
        n311 = event-data() -> ()  [unwired: 1 in, 6 out]
        n312 = Number To Decimal String(number=13) -> (decimal integer string=w335:string)  [unwired: 1 in]
        n313 = Number To Decimal String(number=0) -> (decimal integer string=w336:string)  [unwired: 1 in]
        n314 = TCP Open Connection(remote port or service name=1018, timeout ms (60000)=60000) -> (connection ID=w339:refnum<k5>)  [unwired: 3 in, 1 out]
        n315 = flat-sequence {
          frame #0 {
            n316 = local write "LightSensor"(TRUE) -> ()
            n317 = Wait (ms)(milliseconds to wait=u32 500) -> ()  [unwired: 1 out]
          }
          frame #1 {
            n318 = local write "LightSensor"(FALSE) -> ()
          }
        }
        n319 = Concatenate Strings "Concatenate Strings"(w335, w336) -> (w330:string)
        n320 = local write "Electric"(0.0 ("Electric")) -> ()
        n321 = String Length(string=w330) -> (length=w337:i32)
        n322 = local read "Electric"() -> (w328:dbl)
        n323 = Type Cast(x=w337) -> (*(type *) &x=w329:string)  [unwired: 1 in]
        n324 = TCP Write(connection ID=w339, data in=w329) -> (connection ID out=w340:refnum<k5>, error out=w338:errorcluster)  [unwired: 2 in, 1 out]
        n325 = TCP Write(connection ID=w340, data in=w330, error in (no error)=w338) -> (connection ID out=w341:refnum<k5>)  [unwired: 1 in, 2 out]
        n326 = TCP Close Connection(connection ID=w341) -> ()  [unwired: 2 in, 2 out]
        n327 = property on="Electric" class="DigNum (strict)"("Val(Sgnl)"=w328) -> ()  [unwired: 2 in, 2 out]
      }
      event "OpenD": Value Change {
        n328 = event-data() -> ()  [unwired: 1 in, 6 out]
        n329 = Number To Decimal String(number=47) -> (decimal integer string=w355:string)  [unwired: 1 in]
        n330 = Number To Decimal String(number=0) -> (decimal integer string=w356:string)  [unwired: 1 in]
        n331 = TCP Open Connection(remote port or service name=1018, timeout ms (60000)=60000) -> (connection ID=w359:refnum<k5>)  [unwired: 3 in, 1 out]
        n332 = flat-sequence {
          frame #0 {
            n333 = local write "LightSensor"(TRUE) -> ()
            n334 = Wait (ms)(milliseconds to wait=u32 500) -> ()  [unwired: 1 out]
          }
          frame #1 {
            n335 = local write "LightSensor"(FALSE) -> ()
          }
        }
        n336 = local read "Electric"() -> (w347:dbl)
        n337 = Concatenate Strings "Concatenate Strings"(w355, w356) -> (w350:string)
        n338 = Add(x=w347, y=12.0) -> (x+y=w346:dbl)
        n339 = local write "Electric"(w346) -> ()
        n340 = String Length(string=w350) -> (length=w357:i32)
        n341 = Type Cast(x=w357) -> (*(type *) &x=w349:string)  [unwired: 1 in]
        n342 = TCP Write(connection ID=w359, data in=w349) -> (connection ID out=w360:refnum<k5>, error out=w358:errorcluster)  [unwired: 2 in, 1 out]
        n343 = TCP Write(connection ID=w360, data in=w350, error in (no error)=w358) -> (connection ID out=w361:refnum<k5>)  [unwired: 1 in, 2 out]
        n344 = local read "Electric"() -> (w345:dbl)
        n345 = TCP Close Connection(connection ID=w361) -> ()  [unwired: 2 in, 2 out]
        n346 = property on="Electric" class="DigNum (strict)"("Val(Sgnl)"=w345) -> ()  [unwired: 2 in, 2 out]
      }
      event "Bedroom1DO": Value Change {
        n347 = event-data() -> ()  [unwired: 1 in, 6 out]
        n348 = Number To Decimal String(number=14) -> (decimal integer string=w371:string)  [unwired: 1 in]
        n349 = Number To Decimal String(number=0) -> (decimal integer string=w372:string)  [unwired: 1 in]
        n350 = TCP Open Connection(remote port or service name=1018, timeout ms (60000)=60000) -> (connection ID=w375:refnum<k5>)  [unwired: 3 in, 1 out]
        n351 = flat-sequence {
          frame #0 {
            n352 = local write "DoorSensor"(TRUE) -> ()
            n353 = Wait (ms)(milliseconds to wait=u32 500) -> ()  [unwired: 1 out]
          }
          frame #1 {
            n354 = local write "DoorSensor"(FALSE) -> ()
          }
        }
        n355 = Concatenate Strings "Concatenate Strings"(w371, w372) -> (w366:string)
        n356 = String Length(string=w366) -> (length=w373:i32)
        n357 = Type Cast(x=w373) -> (*(type *) &x=w365:string)  [unwired: 1 in]
        n358 = TCP Write(connection ID=w375, data in=w365) -> (connection ID out=w376:refnum<k5>, error out=w374:errorcluster)  [unwired: 2 in, 1 out]
        n359 = TCP Write(connection ID=w376, data in=w366, error in (no error)=w374) -> (connection ID out=w377:refnum<k5>)  [unwired: 1 in, 2 out]
        n360 = TCP Close Connection(connection ID=w377) -> ()  [unwired: 2 in, 2 out]
      }
      event "Bedroom1DC": Value Change {
        n361 = event-data() -> ()  [unwired: 1 in, 6 out]
        n362 = Number To Decimal String(number=15) -> (decimal integer string=w387:string)  [unwired: 1 in]
        n363 = Number To Decimal String(number=0) -> (decimal integer string=w388:string)  [unwired: 1 in]
        n364 = TCP Open Connection(remote port or service name=1018, timeout ms (60000)=60000) -> (connection ID=w391:refnum<k5>)  [unwired: 3 in, 1 out]
        n365 = flat-sequence {
          frame #0 {
            n366 = local write "DoorSensor"(TRUE) -> ()
            n367 = Wait (ms)(milliseconds to wait=u32 500) -> ()  [unwired: 1 out]
          }
          frame #1 {
            n368 = local write "DoorSensor"(FALSE) -> ()
          }
        }
        n369 = Concatenate Strings "Concatenate Strings"(w387, w388) -> (w382:string)
        n370 = String Length(string=w382) -> (length=w389:i32)
        n371 = Type Cast(x=w389) -> (*(type *) &x=w381:string)  [unwired: 1 in]
        n372 = TCP Write(connection ID=w391, data in=w381) -> (connection ID out=w392:refnum<k5>, error out=w390:errorcluster)  [unwired: 2 in, 1 out]
        n373 = TCP Write(connection ID=w392, data in=w382, error in (no error)=w390) -> (connection ID out=w393:refnum<k5>)  [unwired: 1 in, 2 out]
        n374 = TCP Close Connection(connection ID=w393) -> ()  [unwired: 2 in, 2 out]
      }
      event "Bedroom2DO": Value Change {
        n375 = event-data() -> ()  [unwired: 1 in, 6 out]
        n376 = Number To Decimal String(number=16) -> (decimal integer string=w403:string)  [unwired: 1 in]
        n377 = Number To Decimal String(number=0) -> (decimal integer string=w404:string)  [unwired: 1 in]
        n378 = TCP Open Connection(remote port or service name=1018, timeout ms (60000)=60000) -> (connection ID=w407:refnum<k5>)  [unwired: 3 in, 1 out]
        n379 = flat-sequence {
          frame #0 {
            n380 = local write "DoorSensor"(TRUE) -> ()
            n381 = Wait (ms)(milliseconds to wait=u32 500) -> ()  [unwired: 1 out]
          }
          frame #1 {
            n382 = local write "DoorSensor"(FALSE) -> ()
          }
        }
        n383 = Concatenate Strings "Concatenate Strings"(w403, w404) -> (w398:string)
        n384 = String Length(string=w398) -> (length=w405:i32)
        n385 = Type Cast(x=w405) -> (*(type *) &x=w397:string)  [unwired: 1 in]
        n386 = TCP Write(connection ID=w407, data in=w397) -> (connection ID out=w408:refnum<k5>, error out=w406:errorcluster)  [unwired: 2 in, 1 out]
        n387 = TCP Write(connection ID=w408, data in=w398, error in (no error)=w406) -> (connection ID out=w409:refnum<k5>)  [unwired: 1 in, 2 out]
        n388 = TCP Close Connection(connection ID=w409) -> ()  [unwired: 2 in, 2 out]
      }
      event "Bedroom2DC": Value Change {
        n389 = event-data() -> ()  [unwired: 1 in, 6 out]
        n390 = Number To Decimal String(number=17) -> (decimal integer string=w419:string)  [unwired: 1 in]
        n391 = Number To Decimal String(number=0) -> (decimal integer string=w420:string)  [unwired: 1 in]
        n392 = TCP Open Connection(remote port or service name=1018, timeout ms (60000)=60000) -> (connection ID=w423:refnum<k5>)  [unwired: 3 in, 1 out]
        n393 = flat-sequence {
          frame #0 {
            n394 = local write "DoorSensor"(TRUE) -> ()
            n395 = Wait (ms)(milliseconds to wait=u32 500) -> ()  [unwired: 1 out]
          }
          frame #1 {
            n396 = local write "DoorSensor"(FALSE) -> ()
          }
        }
        n397 = Concatenate Strings "Concatenate Strings"(w419, w420) -> (w414:string)
        n398 = String Length(string=w414) -> (length=w421:i32)
        n399 = Type Cast(x=w421) -> (*(type *) &x=w413:string)  [unwired: 1 in]
        n400 = TCP Write(connection ID=w423, data in=w413) -> (connection ID out=w424:refnum<k5>, error out=w422:errorcluster)  [unwired: 2 in, 1 out]
        n401 = TCP Write(connection ID=w424, data in=w414, error in (no error)=w422) -> (connection ID out=w425:refnum<k5>)  [unwired: 1 in, 2 out]
        n402 = TCP Close Connection(connection ID=w425) -> ()  [unwired: 2 in, 2 out]
      }
      event "LivingRoomDO": Value Change {
        n403 = event-data() -> ()  [unwired: 1 in, 6 out]
        n404 = Number To Decimal String(number=18) -> (decimal integer string=w435:string)  [unwired: 1 in]
        n405 = Number To Decimal String(number=0) -> (decimal integer string=w436:string)  [unwired: 1 in]
        n406 = TCP Open Connection(remote port or service name=1018, timeout ms (60000)=60000) -> (connection ID=w439:refnum<k5>)  [unwired: 3 in, 1 out]
        n407 = flat-sequence {
          frame #0 {
            n408 = local write "DoorSensor"(TRUE) -> ()
            n409 = Wait (ms)(milliseconds to wait=u32 500) -> ()  [unwired: 1 out]
          }
          frame #1 {
            n410 = local write "DoorSensor"(FALSE) -> ()
          }
        }
        n411 = Concatenate Strings "Concatenate Strings"(w435, w436) -> (w430:string)
        n412 = String Length(string=w430) -> (length=w437:i32)
        n413 = Type Cast(x=w437) -> (*(type *) &x=w429:string)  [unwired: 1 in]
        n414 = TCP Write(connection ID=w439, data in=w429) -> (connection ID out=w440:refnum<k5>, error out=w438:errorcluster)  [unwired: 2 in, 1 out]
        n415 = TCP Write(connection ID=w440, data in=w430, error in (no error)=w438) -> (connection ID out=w441:refnum<k5>)  [unwired: 1 in, 2 out]
        n416 = TCP Close Connection(connection ID=w441) -> ()  [unwired: 2 in, 2 out]
      }
      event "LivingRoomDC": Value Change {
        n417 = event-data() -> ()  [unwired: 1 in, 6 out]
        n418 = Number To Decimal String(number=19) -> (decimal integer string=w451:string)  [unwired: 1 in]
        n419 = Number To Decimal String(number=0) -> (decimal integer string=w452:string)  [unwired: 1 in]
        n420 = TCP Open Connection(remote port or service name=1018, timeout ms (60000)=60000) -> (connection ID=w455:refnum<k5>)  [unwired: 3 in, 1 out]
        n421 = flat-sequence {
          frame #0 {
            n422 = local write "DoorSensor"(TRUE) -> ()
            n423 = Wait (ms)(milliseconds to wait=u32 500) -> ()  [unwired: 1 out]
          }
          frame #1 {
            n424 = local write "DoorSensor"(FALSE) -> ()
          }
        }
        n425 = Concatenate Strings "Concatenate Strings"(w451, w452) -> (w446:string)
        n426 = String Length(string=w446) -> (length=w453:i32)
        n427 = Type Cast(x=w453) -> (*(type *) &x=w445:string)  [unwired: 1 in]
        n428 = TCP Write(connection ID=w455, data in=w445) -> (connection ID out=w456:refnum<k5>, error out=w454:errorcluster)  [unwired: 2 in, 1 out]
        n429 = TCP Write(connection ID=w456, data in=w446, error in (no error)=w454) -> (connection ID out=w457:refnum<k5>)  [unwired: 1 in, 2 out]
        n430 = TCP Close Connection(connection ID=w457) -> ()  [unwired: 2 in, 2 out]
      }
      event "LRToiletDO": Value Change {
        n431 = event-data() -> ()  [unwired: 1 in, 6 out]
        n432 = Number To Decimal String(number=20) -> (decimal integer string=w467:string)  [unwired: 1 in]
        n433 = Number To Decimal String(number=0) -> (decimal integer string=w468:string)  [unwired: 1 in]
        n434 = TCP Open Connection(remote port or service name=1018, timeout ms (60000)=60000) -> (connection ID=w471:refnum<k5>)  [unwired: 3 in, 1 out]
        n435 = flat-sequence {
          frame #0 {
            n436 = local write "DoorSensor"(TRUE) -> ()
            n437 = Wait (ms)(milliseconds to wait=u32 500) -> ()  [unwired: 1 out]
          }
          frame #1 {
            n438 = local write "DoorSensor"(FALSE) -> ()
          }
        }
        n439 = Concatenate Strings "Concatenate Strings"(w467, w468) -> (w462:string)
        n440 = String Length(string=w462) -> (length=w469:i32)
        n441 = Type Cast(x=w469) -> (*(type *) &x=w461:string)  [unwired: 1 in]
        n442 = TCP Write(connection ID=w471, data in=w461) -> (connection ID out=w472:refnum<k5>, error out=w470:errorcluster)  [unwired: 2 in, 1 out]
        n443 = TCP Write(connection ID=w472, data in=w462, error in (no error)=w470) -> (connection ID out=w473:refnum<k5>)  [unwired: 1 in, 2 out]
        n444 = TCP Close Connection(connection ID=w473) -> ()  [unwired: 2 in, 2 out]
      }
      event "LRToiletDC": Value Change {
        n445 = event-data() -> ()  [unwired: 1 in, 6 out]
        n446 = Number To Decimal String(number=21) -> (decimal integer string=w483:string)  [unwired: 1 in]
        n447 = Number To Decimal String(number=0) -> (decimal integer string=w484:string)  [unwired: 1 in]
        n448 = TCP Open Connection(remote port or service name=1018, timeout ms (60000)=60000) -> (connection ID=w487:refnum<k5>)  [unwired: 3 in, 1 out]
        n449 = flat-sequence {
          frame #0 {
            n450 = local write "DoorSensor"(TRUE) -> ()
            n451 = Wait (ms)(milliseconds to wait=u32 500) -> ()  [unwired: 1 out]
          }
          frame #1 {
            n452 = local write "DoorSensor"(FALSE) -> ()
          }
        }
        n453 = Concatenate Strings "Concatenate Strings"(w483, w484) -> (w478:string)
        n454 = String Length(string=w478) -> (length=w485:i32)
        n455 = Type Cast(x=w485) -> (*(type *) &x=w477:string)  [unwired: 1 in]
        n456 = TCP Write(connection ID=w487, data in=w477) -> (connection ID out=w488:refnum<k5>, error out=w486:errorcluster)  [unwired: 2 in, 1 out]
        n457 = TCP Write(connection ID=w488, data in=w478, error in (no error)=w486) -> (connection ID out=w489:refnum<k5>)  [unwired: 1 in, 2 out]
        n458 = TCP Close Connection(connection ID=w489) -> ()  [unwired: 2 in, 2 out]
      }
      event "MasterBedroomDO": Value Change {
        n459 = event-data() -> ()  [unwired: 1 in, 6 out]
        n460 = Number To Decimal String(number=22) -> (decimal integer string=w499:string)  [unwired: 1 in]
        n461 = Number To Decimal String(number=0) -> (decimal integer string=w500:string)  [unwired: 1 in]
        n462 = TCP Open Connection(remote port or service name=1018, timeout ms (60000)=60000) -> (connection ID=w503:refnum<k5>)  [unwired: 3 in, 1 out]
        n463 = flat-sequence {
          frame #0 {
            n464 = local write "DoorSensor"(TRUE) -> ()
            n465 = Wait (ms)(milliseconds to wait=u32 500) -> ()  [unwired: 1 out]
          }
          frame #1 {
            n466 = local write "DoorSensor"(FALSE) -> ()
          }
        }
        n467 = Concatenate Strings "Concatenate Strings"(w499, w500) -> (w494:string)
        n468 = String Length(string=w494) -> (length=w501:i32)
        n469 = Type Cast(x=w501) -> (*(type *) &x=w493:string)  [unwired: 1 in]
        n470 = TCP Write(connection ID=w503, data in=w493) -> (connection ID out=w504:refnum<k5>, error out=w502:errorcluster)  [unwired: 2 in, 1 out]
        n471 = TCP Write(connection ID=w504, data in=w494, error in (no error)=w502) -> (connection ID out=w505:refnum<k5>)  [unwired: 1 in, 2 out]
        n472 = TCP Close Connection(connection ID=w505) -> ()  [unwired: 2 in, 2 out]
      }
      event "MasterBedroomDC": Value Change {
        n473 = event-data() -> ()  [unwired: 1 in, 6 out]
        n474 = Number To Decimal String(number=23) -> (decimal integer string=w515:string)  [unwired: 1 in]
        n475 = Number To Decimal String(number=0) -> (decimal integer string=w516:string)  [unwired: 1 in]
        n476 = TCP Open Connection(remote port or service name=1018, timeout ms (60000)=60000) -> (connection ID=w519:refnum<k5>)  [unwired: 3 in, 1 out]
        n477 = flat-sequence {
          frame #0 {
            n478 = local write "DoorSensor"(TRUE) -> ()
            n479 = Wait (ms)(milliseconds to wait=u32 500) -> ()  [unwired: 1 out]
          }
          frame #1 {
            n480 = local write "DoorSensor"(FALSE) -> ()
          }
        }
        n481 = Concatenate Strings "Concatenate Strings"(w515, w516) -> (w510:string)
        n482 = String Length(string=w510) -> (length=w517:i32)
        n483 = Type Cast(x=w517) -> (*(type *) &x=w509:string)  [unwired: 1 in]
        n484 = TCP Write(connection ID=w519, data in=w509) -> (connection ID out=w520:refnum<k5>, error out=w518:errorcluster)  [unwired: 2 in, 1 out]
        n485 = TCP Write(connection ID=w520, data in=w510, error in (no error)=w518) -> (connection ID out=w521:refnum<k5>)  [unwired: 1 in, 2 out]
        n486 = TCP Close Connection(connection ID=w521) -> ()  [unwired: 2 in, 2 out]
      }
      event "MBToiletDO": Value Change {
        n487 = event-data() -> ()  [unwired: 1 in, 6 out]
        n488 = Number To Decimal String(number=24) -> (decimal integer string=w531:string)  [unwired: 1 in]
        n489 = Number To Decimal String(number=0) -> (decimal integer string=w532:string)  [unwired: 1 in]
        n490 = TCP Open Connection(remote port or service name=1018, timeout ms (60000)=60000) -> (connection ID=w535:refnum<k5>)  [unwired: 3 in, 1 out]
        n491 = flat-sequence {
          frame #0 {
            n492 = local write "DoorSensor"(TRUE) -> ()
            n493 = Wait (ms)(milliseconds to wait=u32 500) -> ()  [unwired: 1 out]
          }
          frame #1 {
            n494 = local write "DoorSensor"(FALSE) -> ()
          }
        }
        n495 = Concatenate Strings "Concatenate Strings"(w531, w532) -> (w526:string)
        n496 = String Length(string=w526) -> (length=w533:i32)
        n497 = Type Cast(x=w533) -> (*(type *) &x=w525:string)  [unwired: 1 in]
        n498 = TCP Write(connection ID=w535, data in=w525) -> (connection ID out=w536:refnum<k5>, error out=w534:errorcluster)  [unwired: 2 in, 1 out]
        n499 = TCP Write(connection ID=w536, data in=w526, error in (no error)=w534) -> (connection ID out=w537:refnum<k5>)  [unwired: 1 in, 2 out]
        n500 = TCP Close Connection(connection ID=w537) -> ()  [unwired: 2 in, 2 out]
      }
      event "MBToiletDC": Value Change {
        n501 = event-data() -> ()  [unwired: 1 in, 6 out]
        n502 = Number To Decimal String(number=25) -> (decimal integer string=w547:string)  [unwired: 1 in]
        n503 = Number To Decimal String(number=0) -> (decimal integer string=w548:string)  [unwired: 1 in]
        n504 = TCP Open Connection(remote port or service name=1018, timeout ms (60000)=60000) -> (connection ID=w551:refnum<k5>)  [unwired: 3 in, 1 out]
        n505 = flat-sequence {
          frame #0 {
            n506 = local write "DoorSensor"(TRUE) -> ()
            n507 = Wait (ms)(milliseconds to wait=u32 500) -> ()  [unwired: 1 out]
          }
          frame #1 {
            n508 = local write "DoorSensor"(FALSE) -> ()
          }
        }
        n509 = Concatenate Strings "Concatenate Strings"(w547, w548) -> (w542:string)
        n510 = String Length(string=w542) -> (length=w549:i32)
        n511 = Type Cast(x=w549) -> (*(type *) &x=w541:string)  [unwired: 1 in]
        n512 = TCP Write(connection ID=w551, data in=w541) -> (connection ID out=w552:refnum<k5>, error out=w550:errorcluster)  [unwired: 2 in, 1 out]
        n513 = TCP Write(connection ID=w552, data in=w542, error in (no error)=w550) -> (connection ID out=w553:refnum<k5>)  [unwired: 1 in, 2 out]
        n514 = TCP Close Connection(connection ID=w553) -> ()  [unwired: 2 in, 2 out]
      }
      event "KitchenDO": Value Change {
        n515 = event-data() -> ()  [unwired: 1 in, 6 out]
        n516 = Number To Decimal String(number=26) -> (decimal integer string=w563:string)  [unwired: 1 in]
        n517 = Number To Decimal String(number=0) -> (decimal integer string=w564:string)  [unwired: 1 in]
        n518 = TCP Open Connection(remote port or service name=1018, timeout ms (60000)=60000) -> (connection ID=w567:refnum<k5>)  [unwired: 3 in, 1 out]
        n519 = flat-sequence {
          frame #0 {
            n520 = local write "DoorSensor"(TRUE) -> ()
            n521 = Wait (ms)(milliseconds to wait=u32 500) -> ()  [unwired: 1 out]
          }
          frame #1 {
            n522 = local write "DoorSensor"(FALSE) -> ()
          }
        }
        n523 = Concatenate Strings "Concatenate Strings"(w563, w564) -> (w558:string)
        n524 = String Length(string=w558) -> (length=w565:i32)
        n525 = Type Cast(x=w565) -> (*(type *) &x=w557:string)  [unwired: 1 in]
        n526 = TCP Write(connection ID=w567, data in=w557) -> (connection ID out=w568:refnum<k5>, error out=w566:errorcluster)  [unwired: 2 in, 1 out]
        n527 = TCP Write(connection ID=w568, data in=w558, error in (no error)=w566) -> (connection ID out=w569:refnum<k5>)  [unwired: 1 in, 2 out]
        n528 = TCP Close Connection(connection ID=w569) -> ()  [unwired: 2 in, 2 out]
      }
      event "KitchenDC": Value Change {
        n529 = event-data() -> ()  [unwired: 1 in, 6 out]
        n530 = Number To Decimal String(number=27) -> (decimal integer string=w579:string)  [unwired: 1 in]
        n531 = Number To Decimal String(number=0) -> (decimal integer string=w580:string)  [unwired: 1 in]
        n532 = TCP Open Connection(remote port or service name=1018, timeout ms (60000)=60000) -> (connection ID=w583:refnum<k5>)  [unwired: 3 in, 1 out]
        n533 = flat-sequence {
          frame #0 {
            n534 = local write "DoorSensor"(TRUE) -> ()
            n535 = Wait (ms)(milliseconds to wait=u32 500) -> ()  [unwired: 1 out]
          }
          frame #1 {
            n536 = local write "DoorSensor"(FALSE) -> ()
          }
        }
        n537 = Concatenate Strings "Concatenate Strings"(w579, w580) -> (w574:string)
        n538 = String Length(string=w574) -> (length=w581:i32)
        n539 = Type Cast(x=w581) -> (*(type *) &x=w573:string)  [unwired: 1 in]
        n540 = TCP Write(connection ID=w583, data in=w573) -> (connection ID out=w584:refnum<k5>, error out=w582:errorcluster)  [unwired: 2 in, 1 out]
        n541 = TCP Write(connection ID=w584, data in=w574, error in (no error)=w582) -> (connection ID out=w585:refnum<k5>)  [unwired: 1 in, 2 out]
        n542 = TCP Close Connection(connection ID=w585) -> ()  [unwired: 2 in, 2 out]
      }
      event "KitchenToiletDO": Value Change {
        n543 = event-data() -> ()  [unwired: 1 in, 6 out]
        n544 = Number To Decimal String(number=28) -> (decimal integer string=w595:string)  [unwired: 1 in]
        n545 = Number To Decimal String(number=0) -> (decimal integer string=w596:string)  [unwired: 1 in]
        n546 = TCP Open Connection(remote port or service name=1018, timeout ms (60000)=60000) -> (connection ID=w599:refnum<k5>)  [unwired: 3 in, 1 out]
        n547 = flat-sequence {
          frame #0 {
            n548 = local write "DoorSensor"(TRUE) -> ()
            n549 = Wait (ms)(milliseconds to wait=u32 500) -> ()  [unwired: 1 out]
          }
          frame #1 {
            n550 = local write "DoorSensor"(FALSE) -> ()
          }
        }
        n551 = Concatenate Strings "Concatenate Strings"(w595, w596) -> (w590:string)
        n552 = String Length(string=w590) -> (length=w597:i32)
        n553 = Type Cast(x=w597) -> (*(type *) &x=w589:string)  [unwired: 1 in]
        n554 = TCP Write(connection ID=w599, data in=w589) -> (connection ID out=w600:refnum<k5>, error out=w598:errorcluster)  [unwired: 2 in, 1 out]
        n555 = TCP Write(connection ID=w600, data in=w590, error in (no error)=w598) -> (connection ID out=w601:refnum<k5>)  [unwired: 1 in, 2 out]
        n556 = TCP Close Connection(connection ID=w601) -> ()  [unwired: 2 in, 2 out]
      }
      event "KitchenToiletDC": Value Change {
        n557 = event-data() -> ()  [unwired: 1 in, 6 out]
        n558 = Number To Decimal String(number=29) -> (decimal integer string=w611:string)  [unwired: 1 in]
        n559 = Number To Decimal String(number=0) -> (decimal integer string=w612:string)  [unwired: 1 in]
        n560 = TCP Open Connection(remote port or service name=1018, timeout ms (60000)=60000) -> (connection ID=w615:refnum<k5>)  [unwired: 3 in, 1 out]
        n561 = flat-sequence {
          frame #0 {
            n562 = local write "DoorSensor"(TRUE) -> ()
            n563 = Wait (ms)(milliseconds to wait=u32 500) -> ()  [unwired: 1 out]
          }
          frame #1 {
            n564 = local write "DoorSensor"(FALSE) -> ()
          }
        }
        n565 = Concatenate Strings "Concatenate Strings"(w611, w612) -> (w606:string)
        n566 = String Length(string=w606) -> (length=w613:i32)
        n567 = Type Cast(x=w613) -> (*(type *) &x=w605:string)  [unwired: 1 in]
        n568 = TCP Write(connection ID=w615, data in=w605) -> (connection ID out=w616:refnum<k5>, error out=w614:errorcluster)  [unwired: 2 in, 1 out]
        n569 = TCP Write(connection ID=w616, data in=w606, error in (no error)=w614) -> (connection ID out=w617:refnum<k5>)  [unwired: 1 in, 2 out]
        n570 = TCP Close Connection(connection ID=w617) -> ()  [unwired: 2 in, 2 out]
      }
      event "Balcony1DO1": Value Change {
        n571 = event-data() -> ()  [unwired: 1 in, 6 out]
        n572 = Number To Decimal String(number=30) -> (decimal integer string=w627:string)  [unwired: 1 in]
        n573 = Number To Decimal String(number=0) -> (decimal integer string=w628:string)  [unwired: 1 in]
        n574 = TCP Open Connection(remote port or service name=1018, timeout ms (60000)=60000) -> (connection ID=w631:refnum<k5>)  [unwired: 3 in, 1 out]
        n575 = flat-sequence {
          frame #0 {
            n576 = local write "DoorSensor"(TRUE) -> ()
            n577 = Wait (ms)(milliseconds to wait=u32 500) -> ()  [unwired: 1 out]
          }
          frame #1 {
            n578 = local write "DoorSensor"(FALSE) -> ()
          }
        }
        n579 = Concatenate Strings "Concatenate Strings"(w627, w628) -> (w622:string)
        n580 = String Length(string=w622) -> (length=w629:i32)
        n581 = Type Cast(x=w629) -> (*(type *) &x=w621:string)  [unwired: 1 in]
        n582 = TCP Write(connection ID=w631, data in=w621) -> (connection ID out=w632:refnum<k5>, error out=w630:errorcluster)  [unwired: 2 in, 1 out]
        n583 = TCP Write(connection ID=w632, data in=w622, error in (no error)=w630) -> (connection ID out=w633:refnum<k5>)  [unwired: 1 in, 2 out]
        n584 = TCP Close Connection(connection ID=w633) -> ()  [unwired: 2 in, 2 out]
      }
      event "Balcony1DC1": Value Change {
        n585 = event-data() -> ()  [unwired: 1 in, 6 out]
        n586 = Number To Decimal String(number=31) -> (decimal integer string=w643:string)  [unwired: 1 in]
        n587 = Number To Decimal String(number=0) -> (decimal integer string=w644:string)  [unwired: 1 in]
        n588 = TCP Open Connection(remote port or service name=1018, timeout ms (60000)=60000) -> (connection ID=w647:refnum<k5>)  [unwired: 3 in, 1 out]
        n589 = flat-sequence {
          frame #0 {
            n590 = local write "DoorSensor"(TRUE) -> ()
            n591 = Wait (ms)(milliseconds to wait=u32 500) -> ()  [unwired: 1 out]
          }
          frame #1 {
            n592 = local write "DoorSensor"(FALSE) -> ()
          }
        }
        n593 = Concatenate Strings "Concatenate Strings"(w643, w644) -> (w638:string)
        n594 = String Length(string=w638) -> (length=w645:i32)
        n595 = Type Cast(x=w645) -> (*(type *) &x=w637:string)  [unwired: 1 in]
        n596 = TCP Write(connection ID=w647, data in=w637) -> (connection ID out=w648:refnum<k5>, error out=w646:errorcluster)  [unwired: 2 in, 1 out]
        n597 = TCP Write(connection ID=w648, data in=w638, error in (no error)=w646) -> (connection ID out=w649:refnum<k5>)  [unwired: 1 in, 2 out]
        n598 = TCP Close Connection(connection ID=w649) -> ()  [unwired: 2 in, 2 out]
      }
      event "Balcony1DO2": Value Change {
        n599 = event-data() -> ()  [unwired: 1 in, 6 out]
        n600 = Number To Decimal String(number=32) -> (decimal integer string=w659:string)  [unwired: 1 in]
        n601 = Number To Decimal String(number=0) -> (decimal integer string=w660:string)  [unwired: 1 in]
        n602 = TCP Open Connection(remote port or service name=1018, timeout ms (60000)=60000) -> (connection ID=w663:refnum<k5>)  [unwired: 3 in, 1 out]
        n603 = flat-sequence {
          frame #0 {
            n604 = local write "DoorSensor"(TRUE) -> ()
            n605 = Wait (ms)(milliseconds to wait=u32 500) -> ()  [unwired: 1 out]
          }
          frame #1 {
            n606 = local write "DoorSensor"(FALSE) -> ()
          }
        }
        n607 = Concatenate Strings "Concatenate Strings"(w659, w660) -> (w654:string)
        n608 = String Length(string=w654) -> (length=w661:i32)
        n609 = Type Cast(x=w661) -> (*(type *) &x=w653:string)  [unwired: 1 in]
        n610 = TCP Write(connection ID=w663, data in=w653) -> (connection ID out=w664:refnum<k5>, error out=w662:errorcluster)  [unwired: 2 in, 1 out]
        n611 = TCP Write(connection ID=w664, data in=w654, error in (no error)=w662) -> (connection ID out=w665:refnum<k5>)  [unwired: 1 in, 2 out]
        n612 = TCP Close Connection(connection ID=w665) -> ()  [unwired: 2 in, 2 out]
      }
      event "Balcony1DC2": Value Change {
        n613 = event-data() -> ()  [unwired: 1 in, 6 out]
        n614 = Number To Decimal String(number=33) -> (decimal integer string=w675:string)  [unwired: 1 in]
        n615 = Number To Decimal String(number=0) -> (decimal integer string=w676:string)  [unwired: 1 in]
        n616 = TCP Open Connection(remote port or service name=1018, timeout ms (60000)=60000) -> (connection ID=w679:refnum<k5>)  [unwired: 3 in, 1 out]
        n617 = flat-sequence {
          frame #0 {
            n618 = local write "DoorSensor"(TRUE) -> ()
            n619 = Wait (ms)(milliseconds to wait=u32 500) -> ()  [unwired: 1 out]
          }
          frame #1 {
            n620 = local write "DoorSensor"(FALSE) -> ()
          }
        }
        n621 = Concatenate Strings "Concatenate Strings"(w675, w676) -> (w670:string)
        n622 = String Length(string=w670) -> (length=w677:i32)
        n623 = Type Cast(x=w677) -> (*(type *) &x=w669:string)  [unwired: 1 in]
        n624 = TCP Write(connection ID=w679, data in=w669) -> (connection ID out=w680:refnum<k5>, error out=w678:errorcluster)  [unwired: 2 in, 1 out]
        n625 = TCP Write(connection ID=w680, data in=w670, error in (no error)=w678) -> (connection ID out=w681:refnum<k5>)  [unwired: 1 in, 2 out]
        n626 = TCP Close Connection(connection ID=w681) -> ()  [unwired: 2 in, 2 out]
      }
      event "Balcony2DO": Value Change {
        n627 = event-data() -> ()  [unwired: 1 in, 6 out]
        n628 = Number To Decimal String(number=34) -> (decimal integer string=w691:string)  [unwired: 1 in]
        n629 = Number To Decimal String(number=0) -> (decimal integer string=w692:string)  [unwired: 1 in]
        n630 = TCP Open Connection(remote port or service name=1018, timeout ms (60000)=60000) -> (connection ID=w695:refnum<k5>)  [unwired: 3 in, 1 out]
        n631 = flat-sequence {
          frame #0 {
            n632 = local write "DoorSensor"(TRUE) -> ()
            n633 = Wait (ms)(milliseconds to wait=u32 500) -> ()  [unwired: 1 out]
          }
          frame #1 {
            n634 = local write "DoorSensor"(FALSE) -> ()
          }
        }
        n635 = Concatenate Strings "Concatenate Strings"(w691, w692) -> (w686:string)
        n636 = String Length(string=w686) -> (length=w693:i32)
        n637 = Type Cast(x=w693) -> (*(type *) &x=w685:string)  [unwired: 1 in]
        n638 = TCP Write(connection ID=w695, data in=w685) -> (connection ID out=w696:refnum<k5>, error out=w694:errorcluster)  [unwired: 2 in, 1 out]
        n639 = TCP Write(connection ID=w696, data in=w686, error in (no error)=w694) -> (connection ID out=w697:refnum<k5>)  [unwired: 1 in, 2 out]
        n640 = TCP Close Connection(connection ID=w697) -> ()  [unwired: 2 in, 2 out]
      }
      event "Balcony2DC": Value Change {
        n641 = event-data() -> ()  [unwired: 1 in, 6 out]
        n642 = Number To Decimal String(number=35) -> (decimal integer string=w707:string)  [unwired: 1 in]
        n643 = Number To Decimal String(number=0) -> (decimal integer string=w708:string)  [unwired: 1 in]
        n644 = TCP Open Connection(remote port or service name=1018, timeout ms (60000)=60000) -> (connection ID=w711:refnum<k5>)  [unwired: 3 in, 1 out]
        n645 = flat-sequence {
          frame #0 {
            n646 = local write "DoorSensor"(TRUE) -> ()
            n647 = Wait (ms)(milliseconds to wait=u32 500) -> ()  [unwired: 1 out]
          }
          frame #1 {
            n648 = local write "DoorSensor"(FALSE) -> ()
          }
        }
        n649 = Concatenate Strings "Concatenate Strings"(w707, w708) -> (w702:string)
        n650 = String Length(string=w702) -> (length=w709:i32)
        n651 = Type Cast(x=w709) -> (*(type *) &x=w701:string)  [unwired: 1 in]
        n652 = TCP Write(connection ID=w711, data in=w701) -> (connection ID out=w712:refnum<k5>, error out=w710:errorcluster)  [unwired: 2 in, 1 out]
        n653 = TCP Write(connection ID=w712, data in=w702, error in (no error)=w710) -> (connection ID out=w713:refnum<k5>)  [unwired: 1 in, 2 out]
        n654 = TCP Close Connection(connection ID=w713) -> ()  [unwired: 2 in, 2 out]
      }
      event "CloseD": Value Change {
        n655 = event-data() -> ()  [unwired: 1 in, 6 out]
        n656 = Number To Decimal String(number=36) -> (decimal integer string=w723:string)  [unwired: 1 in]
        n657 = Number To Decimal String(number=0) -> (decimal integer string=w724:string)  [unwired: 1 in]
        n658 = TCP Open Connection(remote port or service name=1018, timeout ms (60000)=60000) -> (connection ID=w727:refnum<k5>)  [unwired: 3 in, 1 out]
        n659 = flat-sequence {
          frame #0 {
            n660 = local write "DoorSensor"(TRUE) -> ()
            n661 = Wait (ms)(milliseconds to wait=u32 500) -> ()  [unwired: 1 out]
          }
          frame #1 {
            n662 = local write "DoorSensor"(FALSE) -> ()
          }
        }
        n663 = Concatenate Strings "Concatenate Strings"(w723, w724) -> (w718:string)
        n664 = String Length(string=w718) -> (length=w725:i32)
        n665 = Type Cast(x=w725) -> (*(type *) &x=w717:string)  [unwired: 1 in]
        n666 = TCP Write(connection ID=w727, data in=w717) -> (connection ID out=w728:refnum<k5>, error out=w726:errorcluster)  [unwired: 2 in, 1 out]
        n667 = TCP Write(connection ID=w728, data in=w718, error in (no error)=w726) -> (connection ID out=w729:refnum<k5>)  [unwired: 1 in, 2 out]
        n668 = TCP Close Connection(connection ID=w729) -> ()  [unwired: 2 in, 2 out]
      }
      event "LivingRoomC": Value Change {
        n669 = event-data() -> ()  [unwired: 1 in, 6 out]
        n670 = Number To Decimal String(number=37) -> (decimal integer string=w739:string)  [unwired: 1 in]
        n671 = Number To Decimal String(number="LivingRoomC") -> (decimal integer string=w740:string)  [unwired: 1 in]
        n672 = TCP Open Connection(remote port or service name=1018, timeout ms (60000)=60000) -> (connection ID=w743:refnum<k5>)  [unwired: 3 in, 1 out]
        n673 = Concatenate Strings "Concatenate Strings"(w739, w740) -> (w735:string)
        n674 = String Length(string=w735) -> (length=w741:i32)
        n675 = Type Cast(x=w741) -> (*(type *) &x=w734:string)  [unwired: 1 in]
        n676 = TCP Write(connection ID=w743, data in=w734) -> (connection ID out=w744:refnum<k5>, error out=w742:errorcluster)  [unwired: 2 in, 1 out]
        n677 = TCP Write(connection ID=w744, data in=w735, error in (no error)=w742) -> (connection ID out=w745:refnum<k5>)  [unwired: 1 in, 2 out]
        n678 = TCP Close Connection(connection ID=w745) -> ()  [unwired: 2 in, 2 out]
      }
      event "MasterBedroomC": Value Change {
        n679 = event-data() -> ()  [unwired: 1 in, 6 out]
        n680 = Number To Decimal String(number=38) -> (decimal integer string=w752:string)  [unwired: 1 in]
        n681 = Number To Decimal String(number="MasterBedroomC") -> (decimal integer string=w753:string)  [unwired: 1 in]
        n682 = TCP Open Connection(remote port or service name=1018, timeout ms (60000)=60000) -> (connection ID=w756:refnum<k5>)  [unwired: 3 in, 1 out]
        n683 = Concatenate Strings "Concatenate Strings"(w752, w753) -> (w748:string)
        n684 = String Length(string=w748) -> (length=w754:i32)
        n685 = Type Cast(x=w754) -> (*(type *) &x=w747:string)  [unwired: 1 in]
        n686 = TCP Write(connection ID=w756, data in=w747) -> (connection ID out=w757:refnum<k5>, error out=w755:errorcluster)  [unwired: 2 in, 1 out]
        n687 = TCP Write(connection ID=w757, data in=w748, error in (no error)=w755) -> (connection ID out=w758:refnum<k5>)  [unwired: 1 in, 2 out]
        n688 = TCP Close Connection(connection ID=w758) -> ()  [unwired: 2 in, 2 out]
      }
      event "Power": Value Change {
        n689 = event-data() -> ()  [unwired: 1 in, 6 out]
        n690 = Number To Decimal String(number=39) -> (decimal integer string=w767:string)  [unwired: 1 in]
        n691 = Number To Decimal String(number=0) -> (decimal integer string=w768:string)  [unwired: 1 in]
        n692 = TCP Open Connection(remote port or service name=1018, timeout ms (60000)=60000) -> (connection ID=w771:refnum<k5>)  [unwired: 3 in, 1 out]
        n693 = flat-sequence {
          frame #0 {
            n694 = local write "TVSensor"(TRUE) -> ()
            n695 = Wait (ms)(milliseconds to wait=u32 500) -> ()  [unwired: 1 out]
          }
          frame #1 {
            n696 = local write "TVSensor"(FALSE) -> ()
          }
        }
        n697 = local read "Electric"() -> (w760:dbl)
        n698 = Concatenate Strings "Concatenate Strings"(w767, w768) -> (w763:string)
        n699 = Decrement(x=w760) -> (x-1=w759:dbl)
        n700 = local write "Electric"(w759) -> ()
        n701 = String Length(string=w763) -> (length=w769:i32)
        n702 = Type Cast(x=w769) -> (*(type *) &x=w762:string)  [unwired: 1 in]
        n703 = TCP Write(connection ID=w771, data in=w762) -> (connection ID out=w772:refnum<k5>, error out=w770:errorcluster)  [unwired: 2 in, 1 out]
        n704 = TCP Write(connection ID=w772, data in=w763, error in (no error)=w770) -> (connection ID out=w773:refnum<k5>)  [unwired: 1 in, 2 out]
        n705 = TCP Close Connection(connection ID=w773) -> ()  [unwired: 2 in, 2 out]
      }
      event "Pause": Value Change {
        n706 = event-data() -> ()  [unwired: 1 in, 6 out]
        n707 = Number To Decimal String(number=40) -> (decimal integer string=w783:string)  [unwired: 1 in]
        n708 = Number To Decimal String(number=0) -> (decimal integer string=w784:string)  [unwired: 1 in]
        n709 = TCP Open Connection(remote port or service name=1018, timeout ms (60000)=60000) -> (connection ID=w787:refnum<k5>)  [unwired: 3 in, 1 out]
        n710 = flat-sequence {
          frame #0 {
            n711 = local write "TVSensor"(TRUE) -> ()
            n712 = Wait (ms)(milliseconds to wait=u32 500) -> ()  [unwired: 1 out]
          }
          frame #1 {
            n713 = local write "TVSensor"(FALSE) -> ()
          }
        }
        n714 = Concatenate Strings "Concatenate Strings"(w783, w784) -> (w779:string)
        n715 = String Length(string=w779) -> (length=w785:i32)
        n716 = Type Cast(x=w785) -> (*(type *) &x=w778:string)  [unwired: 1 in]
        n717 = TCP Write(connection ID=w787, data in=w778) -> (connection ID out=w788:refnum<k5>, error out=w786:errorcluster)  [unwired: 2 in, 1 out]
        n718 = TCP Write(connection ID=w788, data in=w779, error in (no error)=w786) -> (connection ID out=w789:refnum<k5>)  [unwired: 1 in, 2 out]
        n719 = TCP Close Connection(connection ID=w789) -> ()  [unwired: 2 in, 2 out]
      }
      event "Channel1": Value Change {
        n720 = event-data() -> ()  [unwired: 1 in, 6 out]
        n721 = Number To Decimal String(number=41) -> (decimal integer string=w799:string)  [unwired: 1 in]
        n722 = Number To Decimal String(number=0) -> (decimal integer string=w800:string)  [unwired: 1 in]
        n723 = TCP Open Connection(remote port or service name=1018, timeout ms (60000)=60000) -> (connection ID=w803:refnum<k5>)  [unwired: 3 in, 1 out]
        n724 = flat-sequence {
          frame #0 {
            n725 = local write "TVSensor"(TRUE) -> ()
            n726 = Wait (ms)(milliseconds to wait=u32 500) -> ()  [unwired: 1 out]
          }
          frame #1 {
            n727 = local write "TVSensor"(FALSE) -> ()
          }
        }
        n728 = Concatenate Strings "Concatenate Strings"(w799, w800) -> (w795:string)
        n729 = String Length(string=w795) -> (length=w801:i32)
        n730 = Type Cast(x=w801) -> (*(type *) &x=w794:string)  [unwired: 1 in]
        n731 = TCP Write(connection ID=w803, data in=w794) -> (connection ID out=w804:refnum<k5>, error out=w802:errorcluster)  [unwired: 2 in, 1 out]
        n732 = TCP Write(connection ID=w804, data in=w795, error in (no error)=w802) -> (connection ID out=w805:refnum<k5>)  [unwired: 1 in, 2 out]
        n733 = TCP Close Connection(connection ID=w805) -> ()  [unwired: 2 in, 2 out]
      }
      event "Channel2": Value Change {
        n734 = event-data() -> ()  [unwired: 1 in, 6 out]
        n735 = Number To Decimal String(number=42) -> (decimal integer string=w815:string)  [unwired: 1 in]
        n736 = Number To Decimal String(number=0) -> (decimal integer string=w816:string)  [unwired: 1 in]
        n737 = TCP Open Connection(remote port or service name=1018, timeout ms (60000)=60000) -> (connection ID=w819:refnum<k5>)  [unwired: 3 in, 1 out]
        n738 = flat-sequence {
          frame #0 {
            n739 = local write "TVSensor"(TRUE) -> ()
            n740 = Wait (ms)(milliseconds to wait=u32 500) -> ()  [unwired: 1 out]
          }
          frame #1 {
            n741 = local write "TVSensor"(FALSE) -> ()
          }
        }
        n742 = Concatenate Strings "Concatenate Strings"(w815, w816) -> (w811:string)
        n743 = String Length(string=w811) -> (length=w817:i32)
        n744 = Type Cast(x=w817) -> (*(type *) &x=w810:string)  [unwired: 1 in]
        n745 = TCP Write(connection ID=w819, data in=w810) -> (connection ID out=w820:refnum<k5>, error out=w818:errorcluster)  [unwired: 2 in, 1 out]
        n746 = TCP Write(connection ID=w820, data in=w811, error in (no error)=w818) -> (connection ID out=w821:refnum<k5>)  [unwired: 1 in, 2 out]
        n747 = TCP Close Connection(connection ID=w821) -> ()  [unwired: 2 in, 2 out]
      }
      event "Channel3": Value Change {
        n748 = event-data() -> ()  [unwired: 1 in, 6 out]
        n749 = Number To Decimal String(number=43) -> (decimal integer string=w831:string)  [unwired: 1 in]
        n750 = Number To Decimal String(number=0) -> (decimal integer string=w832:string)  [unwired: 1 in]
        n751 = TCP Open Connection(remote port or service name=1018, timeout ms (60000)=60000) -> (connection ID=w835:refnum<k5>)  [unwired: 3 in, 1 out]
        n752 = flat-sequence {
          frame #0 {
            n753 = local write "TVSensor"(TRUE) -> ()
            n754 = Wait (ms)(milliseconds to wait=u32 500) -> ()  [unwired: 1 out]
          }
          frame #1 {
            n755 = local write "TVSensor"(FALSE) -> ()
          }
        }
        n756 = Concatenate Strings "Concatenate Strings"(w831, w832) -> (w827:string)
        n757 = String Length(string=w827) -> (length=w833:i32)
        n758 = Type Cast(x=w833) -> (*(type *) &x=w826:string)  [unwired: 1 in]
        n759 = TCP Write(connection ID=w835, data in=w826) -> (connection ID out=w836:refnum<k5>, error out=w834:errorcluster)  [unwired: 2 in, 1 out]
        n760 = TCP Write(connection ID=w836, data in=w827, error in (no error)=w834) -> (connection ID out=w837:refnum<k5>)  [unwired: 1 in, 2 out]
        n761 = TCP Close Connection(connection ID=w837) -> ()  [unwired: 2 in, 2 out]
      }
      event "Play": Value Change {
        n762 = event-data() -> ()  [unwired: 1 in, 6 out]
        n763 = Number To Decimal String(number=44) -> (decimal integer string=w849:string)  [unwired: 1 in]
        n764 = Number To Decimal String(number=0) -> (decimal integer string=w850:string)  [unwired: 1 in]
        n765 = TCP Open Connection(remote port or service name=1018, timeout ms (60000)=60000) -> (connection ID=w853:refnum<k5>)  [unwired: 3 in, 1 out]
        n766 = flat-sequence {
          frame #0 {
            n767 = local write "TVSensor"(TRUE) -> ()
            n768 = Wait (ms)(milliseconds to wait=u32 500) -> ()  [unwired: 1 out]
          }
          frame #1 {
            n769 = local write "TVSensor"(FALSE) -> ()
          }
        }
        n770 = local read "Electric"() -> (w842:dbl)
        n771 = Concatenate Strings "Concatenate Strings"(w849, w850) -> (w845:string)
        n772 = Increment(x=w842) -> (x+1=w841:dbl)
        n773 = local write "Electric"(w841) -> ()
        n774 = String Length(string=w845) -> (length=w851:i32)
        n775 = Type Cast(x=w851) -> (*(type *) &x=w844:string)  [unwired: 1 in]
        n776 = TCP Write(connection ID=w853, data in=w844) -> (connection ID out=w854:refnum<k5>, error out=w852:errorcluster)  [unwired: 2 in, 1 out]
        n777 = TCP Write(connection ID=w854, data in=w845, error in (no error)=w852) -> (connection ID out=w855:refnum<k5>)  [unwired: 1 in, 2 out]
        n778 = TCP Close Connection(connection ID=w855) -> ()  [unwired: 2 in, 2 out]
      }
      event "Volume": Value Change {
        n779 = event-data() -> ()  [unwired: 1 in, 6 out]
        n780 = Number To Decimal String(number=45) -> (decimal integer string=w865:string)  [unwired: 1 in]
        n781 = Number To Decimal String(number="Volume") -> (decimal integer string=w866:string)  [unwired: 1 in]
        n782 = TCP Open Connection(remote port or service name=1018, timeout ms (60000)=60000) -> (connection ID=w869:refnum<k5>)  [unwired: 3 in, 1 out]
        n783 = flat-sequence {
          frame #0 {
            n784 = local write "TVSensor"(TRUE) -> ()
            n785 = Wait (ms)(milliseconds to wait=u32 500) -> ()  [unwired: 1 out]
          }
          frame #1 {
            n786 = local write "TVSensor"(FALSE) -> ()
          }
        }
        n787 = Concatenate Strings "Concatenate Strings"(w865, w866) -> (w861:string)
        n788 = String Length(string=w861) -> (length=w867:i32)
        n789 = Type Cast(x=w867) -> (*(type *) &x=w860:string)  [unwired: 1 in]
        n790 = TCP Write(connection ID=w869, data in=w860) -> (connection ID out=w870:refnum<k5>, error out=w868:errorcluster)  [unwired: 2 in, 1 out]
        n791 = TCP Write(connection ID=w870, data in=w861, error in (no error)=w868) -> (connection ID out=w871:refnum<k5>)  [unwired: 1 in, 2 out]
        n792 = TCP Close Connection(connection ID=w871) -> ()  [unwired: 2 in, 2 out]
      }
      event "Electric": Value Change {
        n793 = event-data() -> ()  [unwired: 1 in, 6 out]
        n794 = flat-sequence {
          tunnel: [w884] -> w875
          tunnel: [w888] -> w876
          tunnel: w875 -> [w887]
          tunnel: w876 -> [w898]
          frame #0 {
            n795 = local read "Electric"() -> (w880:dbl)
            n796 = Less Than 0?(x=w880) -> (x < 0?=w881:bool)
            n797 = local read "Electric"() -> (w879:dbl)
            n798 = Greater?(x=w879, y=12.0) -> (0:w878:bool)
            n799 = case shown="True" w878 {
              frame False {
              }
              frame True {
                n800 = local write "Electric"(12.0 ("Electric")) -> ()
              }
            }
            n801 = case shown="True" w881 {
              frame False {
              }
              frame True {
                n802 = local write "Electric"(0.0 ("Electric")) -> ()
              }
            }
          }
          frame #1 {
            n803 = TCP Open Connection(remote port or service name=1018, timeout ms (60000)=60000) -> (connection ID=w884:refnum<k5>)  [unwired: 3 in, 1 out]
          }
          frame #2 {
            n804 = Number To Decimal String(number=46) -> (decimal integer string=w895:string)  [unwired: 1 in]
            n805 = Number To Decimal String(number="Electric") -> (decimal integer string=w894:string)  [unwired: 1 in]
            n806 = Concatenate Strings "Concatenate Strings"(w895, w894) -> (w896:string)
            n807 = String Length(string=w896) -> (length=w893:i32)
            n808 = Type Cast(x=w893) -> (*(type *) &x=w889:string)  [unwired: 1 in]
            n809 = TCP Write(connection ID=w887, data in=w889) -> (connection ID out=w891:refnum<k5>, error out=w892:errorcluster)  [unwired: 2 in, 1 out]
            n810 = TCP Write(connection ID=w891, data in=w896, error in (no error)=w892) -> (connection ID out=w888:refnum<k5>)  [unwired: 1 in, 2 out]
          }
          frame #3 {
            n811 = TCP Close Connection(connection ID=w898) -> ()  [unwired: 2 in, 2 out]
          }
        }
      }
    }
  }
